vi "EnFlo_Tun_Heater_Control.vi"(1 "Heaters Enabled time (s)":dbl, 2 "Heaters Just Enabled":bool, 3 "Ch Names":string[](array[string]), 4 "Values":dbl[](array[numeric]) format="%.2f") -> (0 "Error String":string)   [LabVIEW 2021]
uses:
  ADAM Client/Sub VIs/ADAM Controls/Search_mode.ctl
  <vilib>/Analysis/baseanly.llb/Mean (DBL).vi
  ADAM_Global.vi
  Anemometry/Anemometry Sub Vis/Globals/EnFlo_Tunnel_Global.vi
  <vilib>/Analysis/NI_AALPro.lvlib
  <vilib>/Analysis/NI_AALBase.lvlib
panel:
  in  "Time (s) before killing heaters when exceeding max power":i32=350
  out "Heater State Happy":bool
  out "Error":dbl(graph)
  out "Derivative":dbl(graph)
  out "Integral":dbl(graph)
  out "Proportional":dbl(graph)
  out "Upper limit on Power":dbl
  in  "Proportional Error Deadband":dbl=0.03
  out "Read Values OK":bool
  out "History Out":dbl[](array[numeric])
  out "Current Temp":dbl
  out "Setpoint":dbl
  in  "Index To Display":i32
  out "Feedback Temperature":string
  in  "Minimum Power Change in %":dbl=0.05
  in  "Total History":i32=450
  out "Control Sum":dbl format="%#.1f"
  in  "Derivative History":i32=60
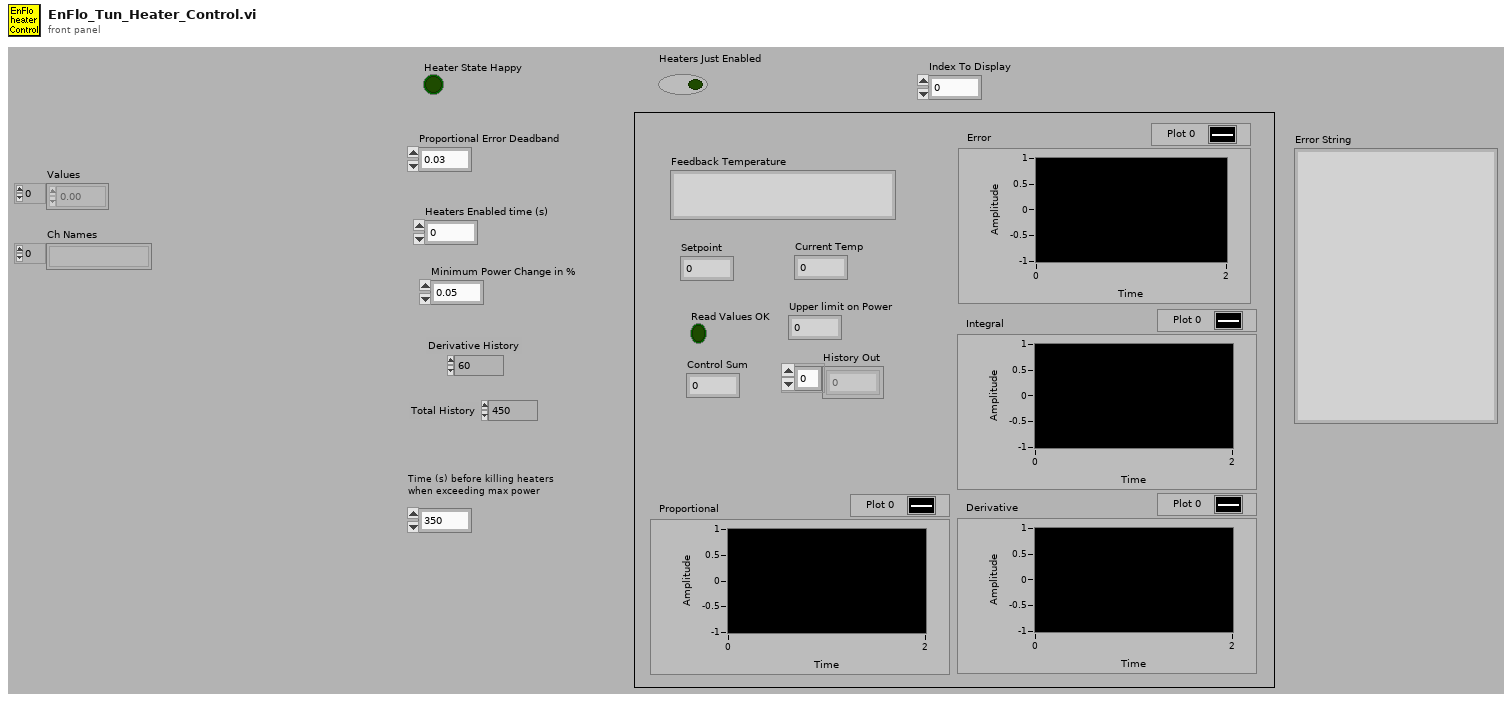
[diagram p1: front panel]
types:
  T1 = enum16{"On", "Off", "Always On", "Always Off", "Delete"}
  T2 = typedef "Search_mode.ctl" = enum16{"Between times", "All Times"}
  T3 = typedef "Ch_description_ADAM.ctl" = cluster{"Ch Name":string, "Type":T4, "Function":T5, "Ch State":T6, "Calibration type":T7, "A":dbl, "B":dbl, "C":dbl, "D":dbl, "Comments":string, "Address":T8, "String":string, "Duty":u16}
  T4 = typedef "Module_type_ADAM.ctl" = string
  T5 = typedef "Function_ADAM.ctl" = enum16{"Analogue Input", "Digital Input", "Event counter", "Event rate", "Analogue Output", "Digital Output", "Relay Output"}
  T6 = typedef "Channel_State.ctl" = enum16{"On", "Off", "Always On", "Always Off"}
  T7 = typedef "Calib_type_ADAM.ctl" = string
  T8 = typedef "Address.ctl" = cluster{"Main":i32, "Ch.":i32, "Sub":i32, "Port Name":string}
  T9 = cluster{"Bus Bar":string, "Connected Items":string[]}
  T10 = cluster{"Bus Bar":string, "Connected Items":string[]}[]
  T11 = cluster{"Centre Times":dbl[], "Output array":dbl[]}
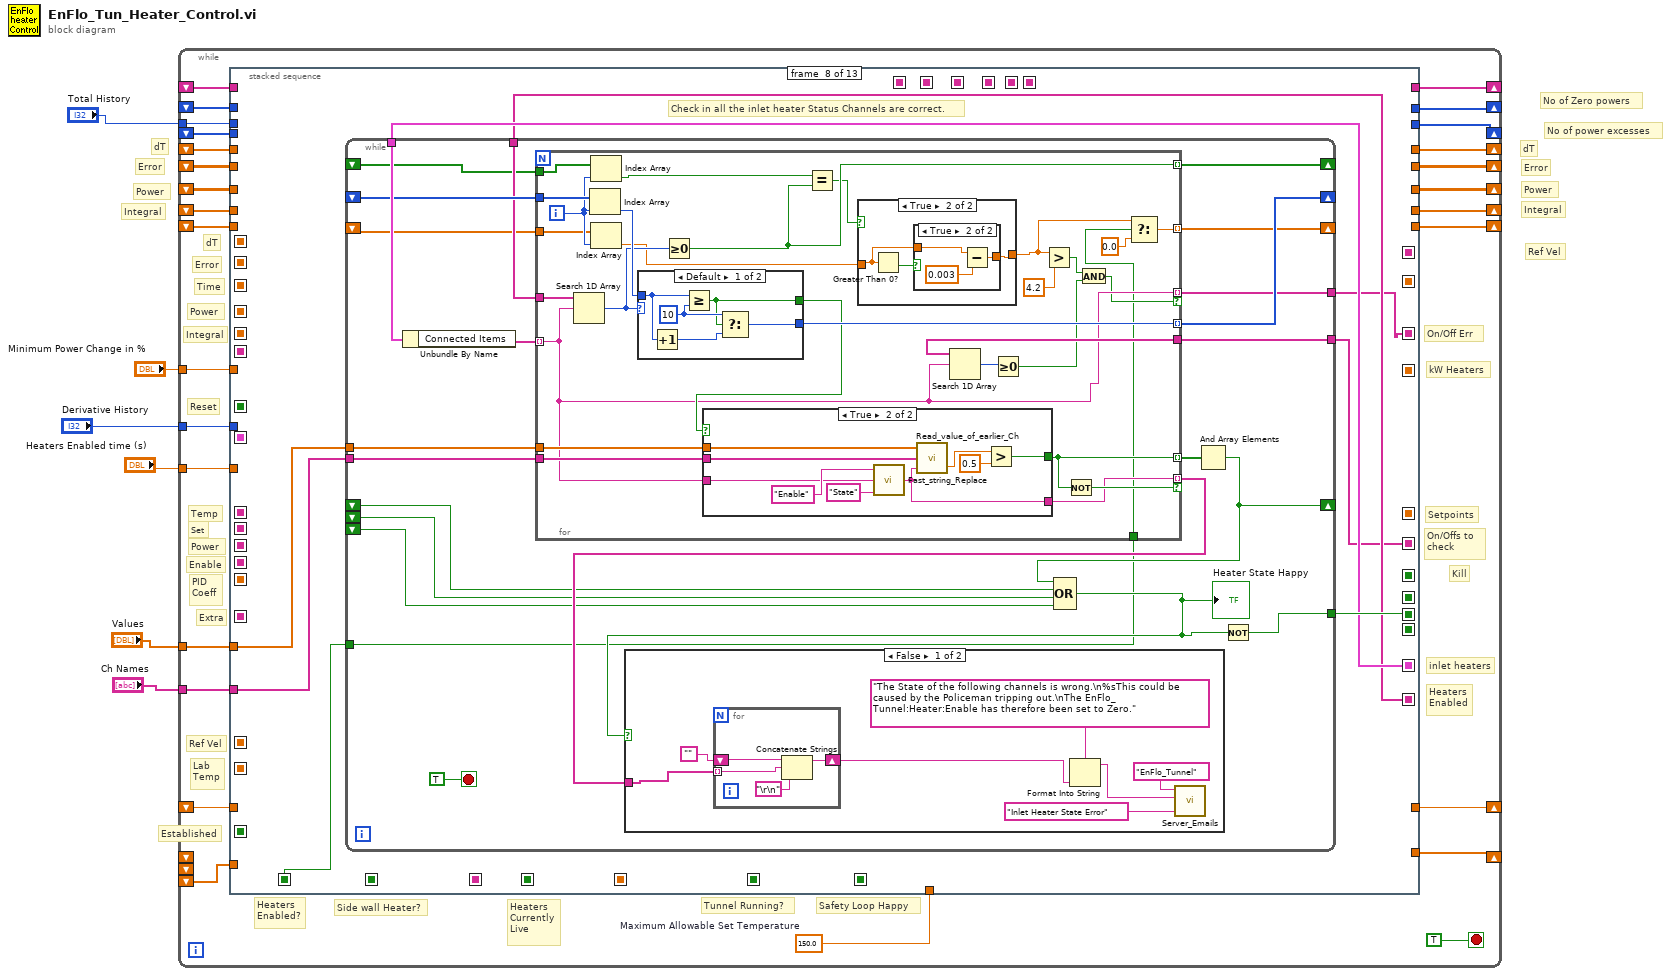
[diagram p0: block diagram]
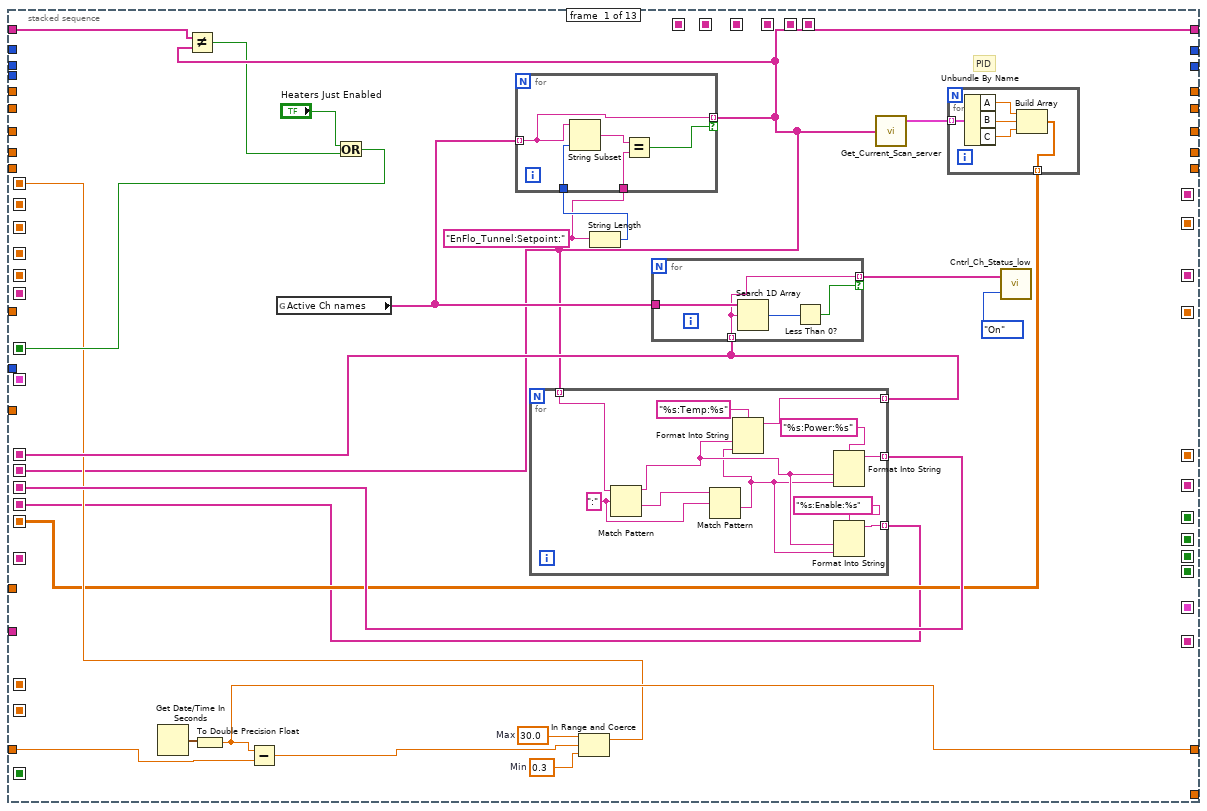
[diagram p2: hidden frame]
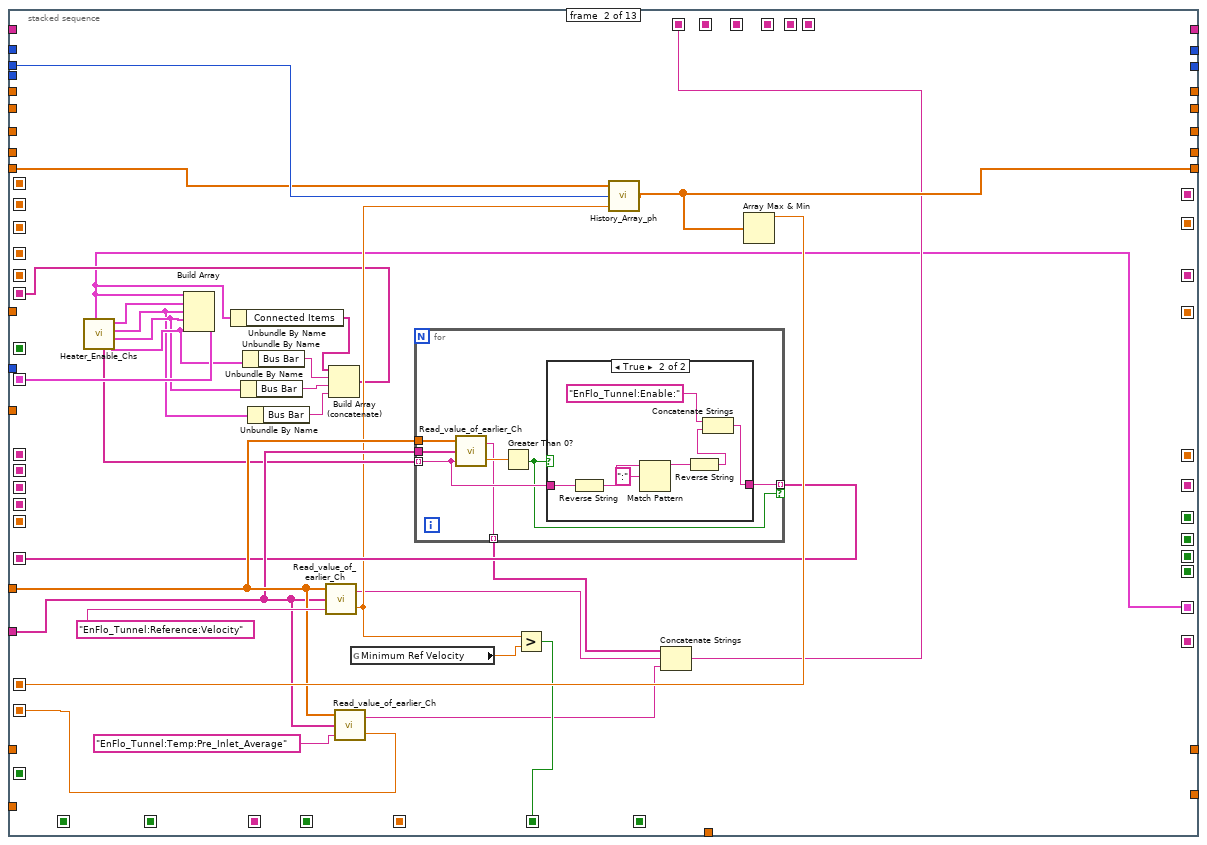
[diagram p3: hidden frame]
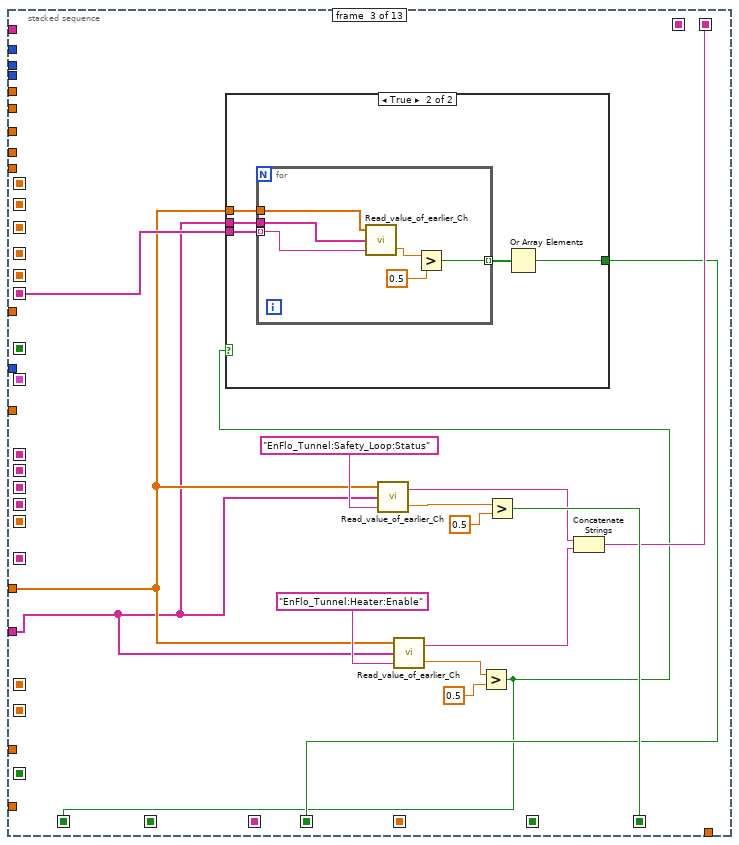
[diagram p5: hidden frame]
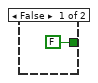
[diagram p6: hidden frame]
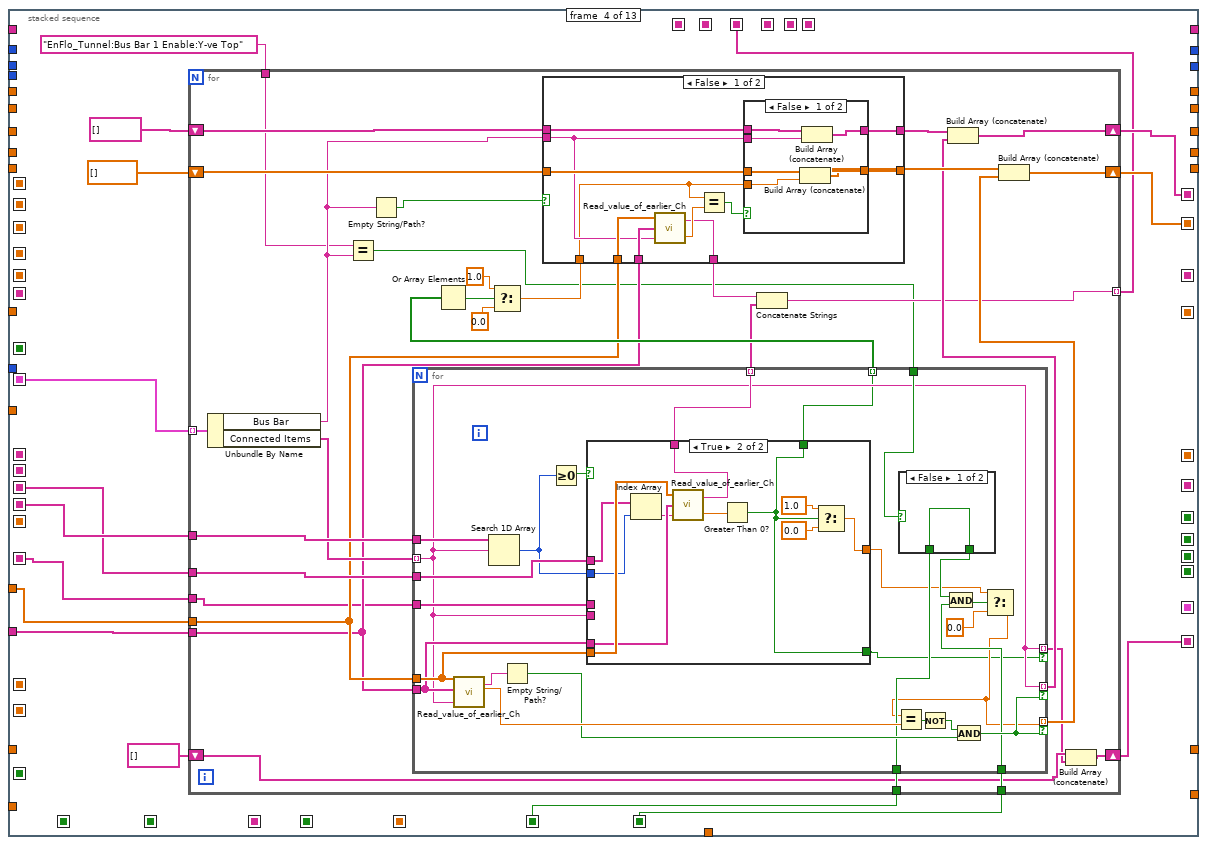
[diagram p7: hidden frame]
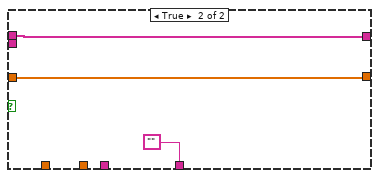
[diagram p9: hidden frame]
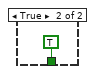
[diagram p10: hidden frame]
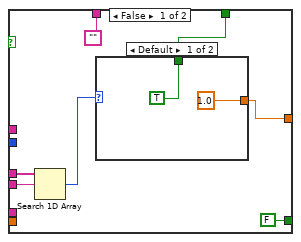
[diagram p11: hidden frame]
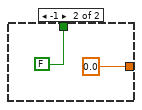
[diagram p12: hidden frame]
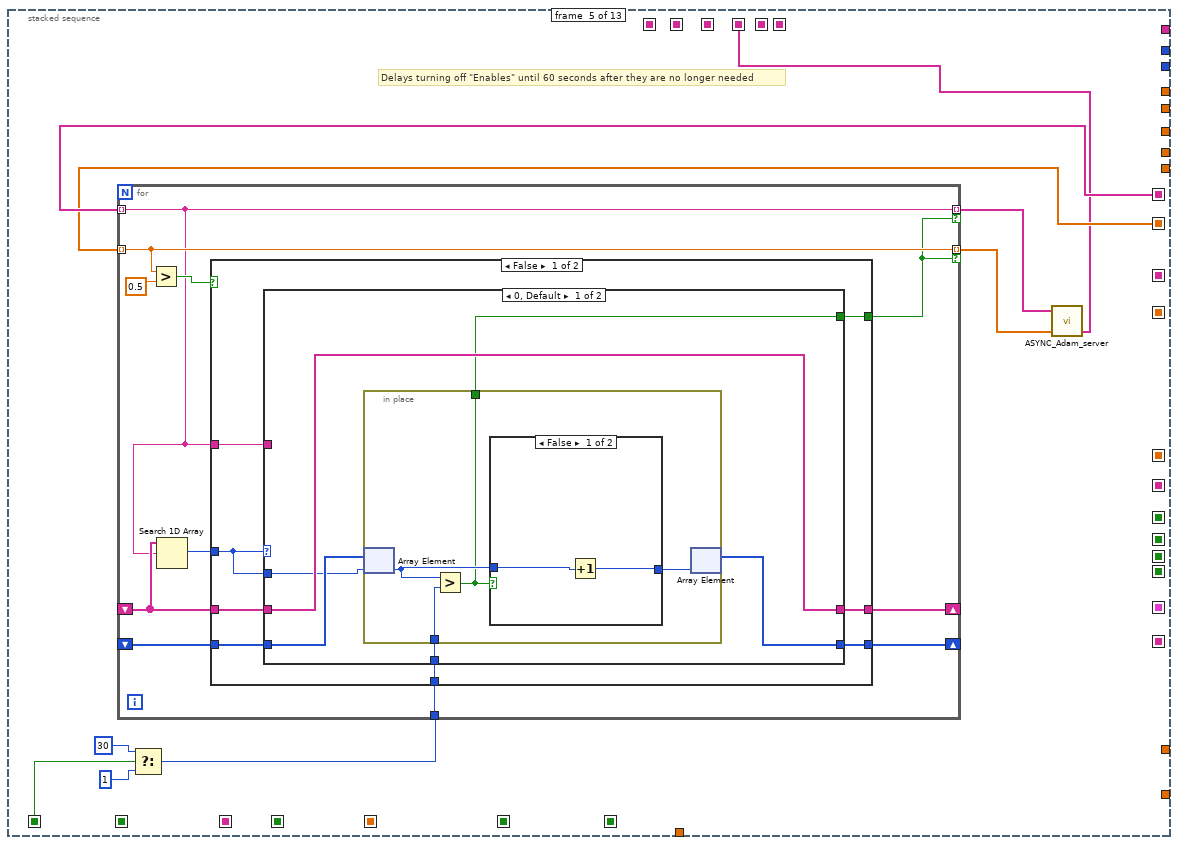
[diagram p13: hidden frame]
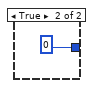
[diagram p14: hidden frame]
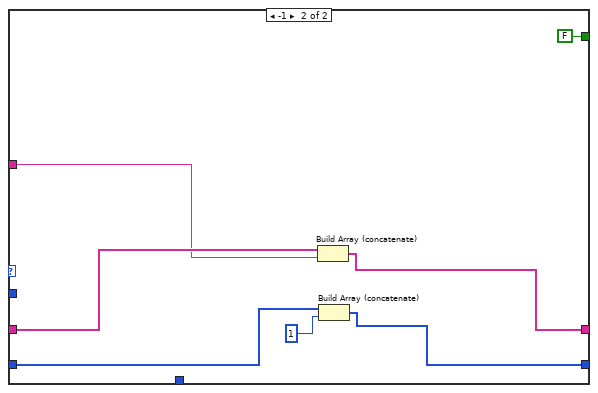
[diagram p15: hidden frame]
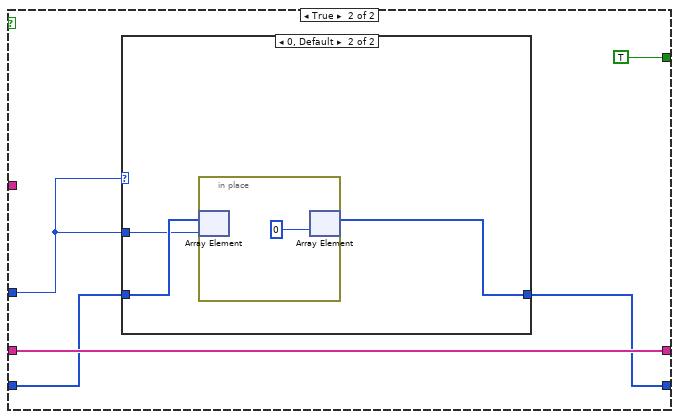
[diagram p16: hidden frame]
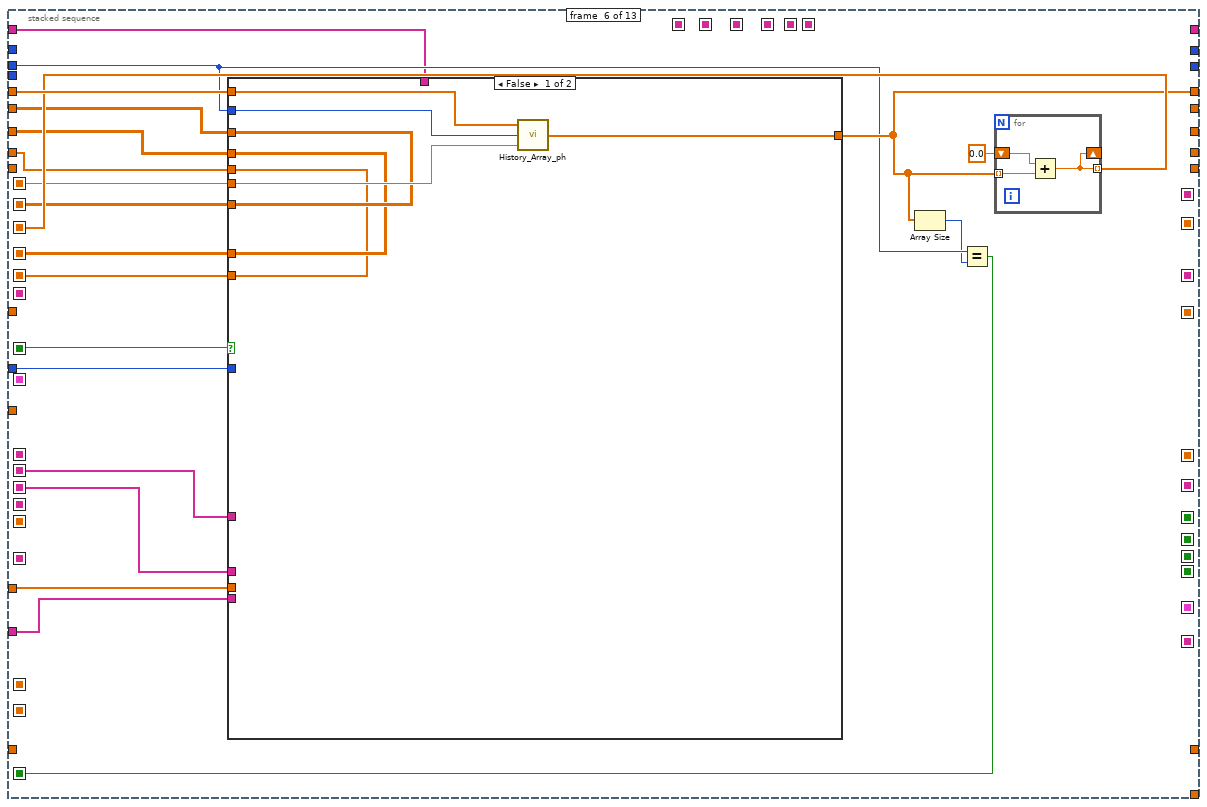
[diagram p18: hidden frame]
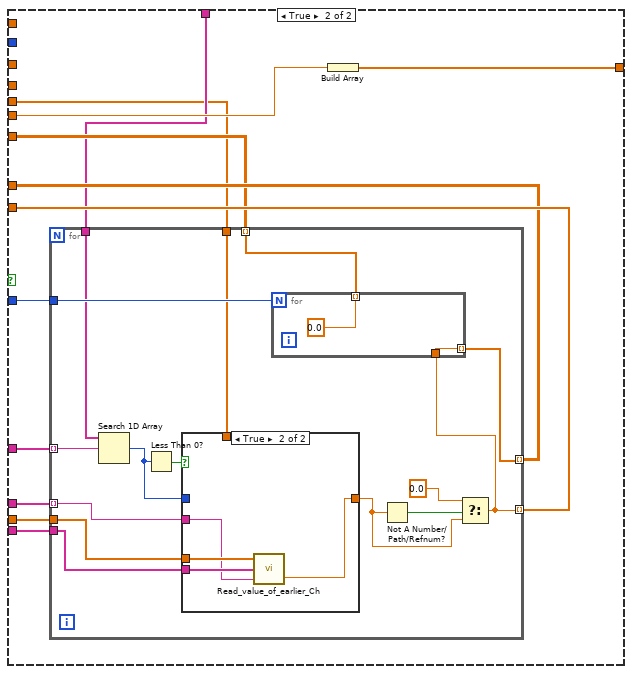
[diagram p19: hidden frame]
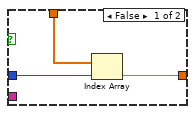
[diagram p20: hidden frame]
diagram:
  # "Established"
  # "No of Zero powers"
  # "No of power excesses"
  # "Ref Vel"
  # "Integral"
  # "Power"
  # "Error"
  # "dT"
  # "Power"
  # "Integral"
  # "Error"
  # "dT"
  n1 = while {
    shift-right: [w32] -> _
    shift-left: _ -> [w33]
    shift-right: [w28] -> _
    shift-left: _ -> [w31]
    shift-right: [w30] -> _
    shift-left: _ -> [w29]
    shift-right: [w26] -> _
    shift-left: _ -> [w27]
    shift-right: [w24] -> _
    shift-left: _ -> [w25]
    tunnel: "Total History" -> [w23]
    tunnel: "Ch Names" -> [w21]
    tunnel: "Values" -> [w20]
    tunnel: "Minimum Power Change in %" -> [w19]
    shift-right: [w18] -> _
    shift-left: _ -> [_]
    shift-left: _ -> [_]
    tunnel: "Heaters Enabled time (s)" -> [w17]
    shift-right: [w15] -> _
    shift-left: _ -> [w16]
    shift-right: [w14] -> _
    shift-left: _ -> [w13]
    shift-right: [w11] -> _
    shift-left: _ -> [w12]
    shift-right: [w10] -> _
    shift-left: _ -> [w9]
    shift-left: _ -> [w8]
    tunnel: "Derivative History" -> [w7]
    stop <- TRUE stop-if-true
    w22 = 150.0  # Maximum Allowable Set Temperature
    # "On/Offs to\ncheck"
    # "On/Off Err"
    # "kW Heaters"
    # "inlet heaters"
    # "Heaters\nEnabled"
    # "Heaters\nCurrently\nLive"
    # "Heaters\nEnabled?"
    # "Safety Loop Happy"
    # "Tunnel Running?"
    # "Setpoints"
    # "Extra"
    # "Enable"
    # "Side wall Heater?"
    # "Lab\nTemp"
    # "Ref Vel"
    # "PID\nCoeff"
    # "dT"
    # "Integral"
    # "Power"
    # "Error"
    # "Reset"
    # "Kill"
    # "Power"
    # "Set"
    # "Temp"
    # "Time"
    n2 = stacked-sequence {
      seq-local: [_ _ _ _ _ w347 _ _ _ _ _ _ _] -> [_ _ _ _ _ _ w433 _ w812 _ _ _ _]
      seq-local: [w47 _ _ _ _ _ _ _ _ _ _ _ _] -> [_ _ _ _ _ _ w430 _ _ _ _ w1028 _]
      seq-local: [w37 _ _ _ _ _ _ _ _ _ _ _ _] -> [_ _ _ _ _ w330 w429 _ _ _ _ w1027 _]
      seq-local: [w54 _ _ _ _ _ _ _ _ _ _ _ _] -> [_ _ _ w165 _ w333 w428 _ _ _ _ w1030 _]
      seq-local: [_ _ _ _ _ _ w413 _ _ _ _ _ _] -> [_ _ _ _ _ _ _ _ w815 _ _ _ _]
      seq-local: [_ _ _ _ _ _ _ _ w814 _ _ _ _] -> [_ _ _ _ _ _ _ _ _ _ _ _ w1110]
      seq-local: [_ _ _ _ _ _ _ _ _ _ w954 _ _] -> [_ _ _ _ _ _ _ _ _ _ _ _ w1111]
      seq-local: [w42 _ _ _ _ _ _ _ _ _ _ _ _] -> [_ _ _ _ _ w346 w424 _ _ _ _ _ _]
      seq-local: [w43 _ _ _ _ _ _ _ _ _ _ _ _] -> [_ _ _ _ _ w349 _ _ _ _ _ w1013 _]
      seq-local: [_ _ _ _ _ w345 _ _ _ _ _ _ _] -> [_ _ _ _ _ _ w421 _ _ _ _ _ _]
      seq-local: [_ _ _ _ _ w343 _ _ _ _ _ _ _] -> [_ _ _ _ _ _ w422 _ _ _ _ _ _]
      seq-local: [_ _ _ _ _ w341 _ _ _ _ _ _ _] -> [_ _ _ _ _ _ w423 _ _ _ _ _ _]
      seq-local: [w40 _ _ _ _ _ _ _ _ _ _ _ _] -> [_ _ _ _ _ _ w419 _ _ _ _ _ _]
      seq-local: [_ _ _ _ _ w337 _ _ _ _ _ _ _] -> [_ _ _ _ _ _ _ _ _ _ _ w1007 _]
      seq-local: [_ w104 _ _ _ _ _ _ _ _ _ _ _] -> [_ _ _ _ _ _ w415 _ _ _ _ w1010 _]
      seq-local: [_ w108 _ _ _ _ _ _ _ _ _ _ _] -> [_ _ _ _ _ _ w414 _ _ _ _ _ _]
      seq-local: [_ _ _ _ _ _ w412 _ _ _ _ _ _] -> [_ _ _ _ _ _ _ _ w813 _ _ _ _]
      seq-local: [_ _ _ _ _ _ w411 _ _ _ _ _ _] -> [_ _ _ _ _ _ _ _ _ _ _ w1014 _]
      seq-local: [w38 _ _ _ _ _ _ _ _ _ _ _ _] -> [_ _ _ w166 _ _ w402 _ _ _ _ _ _]
      seq-local: [_ w103 _ _ _ _ _ _ _ _ _ _ _] -> [_ _ _ w162 _ _ _ _ _ _ _ _ _]
      seq-local: [_ w99 _ _ _ _ _ _ _ _ _ _ _] -> [_ _ _ w161 _ _ _ _ _ _ _ _ _]
      seq-local: [_ _ _ w160 _ _ _ _ _ _ _ _ _] -> [_ _ _ _ w280 _ _ _ _ _ _ _ _]
      seq-local: [_ _ _ w159 _ _ _ _ _ _ _ _ _] -> [_ _ _ _ w277 _ _ _ _ _ _ _ _]
      seq-local: [_ _ _ _ _ _ w408 _ _ _ _ _ _] -> [_ _ _ _ _ _ _ _ _ _ w951 _ _]
      seq-local: [_ w96 _ _ _ _ _ _ _ _ _ _ _] -> [_ _ _ w157 _ _ _ _ _ _ _ _ _]
      seq-local: [_ _ w137 _ _ _ _ _ _ _ _ _ _] -> [_ _ _ w156 _ _ _ _ _ _ _ _ _]
      seq-local: [_ w92 _ _ _ _ _ _ _ _ _ _ _] -> [_ _ _ _ _ _ _ _ _ _ _ _ w1115]
      seq-local: [_ _ w131 _ _ _ _ _ _ _ _ _ _] -> [_ _ _ _ _ _ _ _ _ _ _ _ w1116]
      seq-local: [_ _ _ w158 _ _ _ _ _ _ _ _ _] -> [_ _ _ _ _ _ _ _ _ _ _ _ w1117]
      seq-local: [_ _ _ _ w276 _ _ _ _ _ _ _ _] -> [_ _ _ _ _ _ _ _ _ _ _ _ w1118]
      seq-local: [_ _ _ _ _ _ w407 _ _ _ _ _ _] -> [_ _ _ _ _ _ _ _ _ _ _ _ w1119]
      seq-local: [_ _ _ _ _ _ _ _ _ _ _ w1005 _] -> [_ _ _ _ _ _ _ _ _ _ _ _ w1120]
      seq-local: [_ _ w126 _ _ _ _ _ _ _ _ _ _] -> [_ _ _ _ w275 _ w406 w711 w810 _ _ w1004 _]
      seq-local: [_ w84 _ _ _ _ _ _ _ _ _ _ _] -> [_ _ w130 _ _ _ _ _ _ _ _ _ _]
      seq-local: [_ _ w127 _ _ _ _ _ _ _ _ _ _] -> [_ _ _ _ _ _ _ _ _ w934 w949 _ _]
      seq-local: [_ _ _ w153 _ _ _ _ _ _ _ _ _] -> [_ _ _ _ _ _ _ w714 _ _ _ _ _]
      seq-local: [_ _ _ _ _ _ _ w716 _ _ _ _ _] -> [_ _ _ _ _ _ _ _ _ _ _ _ w1112]
      seq-local: [_ w82 _ _ _ _ _ _ _ _ _ _ _] -> [_ _ _ _ _ _ _ w715 _ _ _ _ _]
      seq-local: [_ _ _ _ _ _ _ w713 _ _ _ _ _] -> [_ _ _ _ _ _ _ _ _ w937 _ _ _]
      seq-local: [_ _ _ _ _ _ _ _ _ w933 _ _ _] -> [_ _ _ _ _ _ _ _ _ _ _ _ w1108]
      seq-local: [_ _ _ _ _ _ w404 _ _ _ _ _ _] -> [_ _ _ _ _ _ _ _ _ _ _ _ w1106]
      seq-local: [_ _ _ _ _ _ w403 _ _ _ _ _ _] -> [_ _ _ _ _ _ _ w712 _ _ _ _ _]
      tunnel: w33 -> [_ _ _ _ _ w350 w401 _ _ _ _ _ _]
      tunnel: [_ _ _ _ _ w339 _ _ _ _ _ _ _] -> w32
      tunnel: w31 -> [_ _ _ _ _ w344 _ _ _ _ _ _ _]
      tunnel: [w48 _ _ _ _ _ _ _ _ _ _ _ _] -> w30
      tunnel: w29 -> [w50 _ _ _ _ _ _ _ _ _ _ _ _]
      tunnel: [_ _ _ _ _ _ w434 _ _ _ _ _ _] -> w28
      tunnel: w27 -> [_ _ _ _ _ w342 _ _ _ _ _ w1029 _]
      tunnel: [_ _ _ _ _ _ w432 _ _ _ _ _ _] -> w26
      tunnel: w25 -> [_ _ _ _ _ w340 _ _ _ _ _ _ _]
      tunnel: [_ _ _ _ _ _ w431 _ _ _ _ _ _] -> w24
      tunnel: w23 -> [_ w107 _ _ _ w338 w425 _ w816 _ w955 _ _]
      tunnel: w22 -> [_ _ _ _ _ _ _ _ _ _ w950 _ _]
      tunnel: w21 -> [_ w101 w128 w167 _ w334 w427 w717 _ _ w953 w1025 w1121]
      tunnel: w20 -> [_ w102 w129 w168 _ w335 w426 w718 _ _ w952 w1026 _]
      tunnel: w19 -> [_ _ _ _ _ _ w420 _ _ _ _ w1022 _]
      tunnel: [_ _ _ _ _ _ _ _ _ _ _ w1016 _] -> w18
      tunnel: w8 -> [_ _ _ _ _ _ _ _ _ _ _ w1015 _]
      tunnel: w17 -> [_ _ _ _ _ _ w418 _ _ _ _ _ _]
      tunnel: w16 -> [_ w106 _ _ _ _ _ _ _ _ _ _ _]
      tunnel: [_ w105 _ _ _ _ _ _ _ _ _ _ _] -> w15
      tunnel: [_ _ _ _ _ _ w410 _ _ _ _ _ _] -> w14
      tunnel: w13 -> [_ _ _ _ _ _ w409 _ _ _ _ _ _]
      tunnel: w12 -> [_ _ _ _ _ _ _ _ _ _ _ w1012 _]
      tunnel: [_ _ _ _ _ _ _ _ _ _ _ w1011 _] -> w11
      tunnel: [w37 _ _ _ _ _ _ _ _ _ _ _ _] -> w10
      tunnel: w9 -> [w35 _ _ _ _ w331 _ _ _ _ _ _ _]
      tunnel: w7 -> [_ _ _ _ _ w332 w405 _ _ _ _ _ _]
      frame #0 {
        w52 = 0.3  # Min
        w51 = 30.0  # Max
        w55 = "EnFlo_Tunnel:Setpoint:"
        # "PID"
        n3 = Get Date/Time In Seconds() -> (seconds since 1Jan1904=w53:timestamp)
        n4 = To Double Precision Float(number=w53) -> (double precision float=w48:dbl)
        n5 = Subtract(x=w48, y=w50) -> (x-y=w49:dbl)
        n6 = global read "ADAM_Global.vi" "Active Ch names"() -> (w45:string[])
        n7 = In Range and Coerce(upper limit=w51, x=w49, lower limit=w52) -> (coerced(x)=w42:dbl)  [unwired: 1 out]
        n8 = String Length(string=w55) -> (length=w56:i32)
        n9 = for {
          tunnel: w45 -> [w67] mode=indexing
          tunnel: w56 -> [w70]
          tunnel: w55 -> [w69]
          tunnel: [w67] -> w37 mode=indexing if=w66
          n10 = String Subset(string=w67, length (rest)=w70) -> (substring=w68:string)  [unwired: 1 out]
          n11 = Equal?(x=w68, y=w69) -> (x = y?=w66:bool)
        }
        n12 = Not Equal?(x=w35, y=w37) -> (x != y?=w36:bool)
        n13 = Or(x="Heaters Just Enabled", y=w36) -> (x .or. y?=w43:bool)
        n14 = for {
          tunnel: w37 -> [w75] mode=indexing
          tunnel: [w76] -> w54 mode=indexing
          tunnel: [w77] -> w47 mode=indexing
          tunnel: [w71] -> w38 mode=indexing
          w80 = ":" ("regular expression")
          n15 = Match Pattern(string=w75, regular expression=w80) -> (before substring=w73:string, after substring=w81:string)  [unwired: 3 out]
          n16 = Match Pattern(string=w81, regular expression=w80) -> (after substring=w72:string)  [unwired: 4 out]
          n17 = Format Into String(format string="%s:Temp:%s", w73, w72) -> (resulting string=w77:string)  [unwired: 2 in, 1 out]
          n18 = Format Into String(format string="%s:Power:%s", w73, w72) -> (resulting string=w76:string)  [unwired: 2 in, 1 out]
          n19 = Format Into String(format string="%s:Enable:%s", w73, w72) -> (resulting string=w71:string)  [unwired: 2 in, 1 out]
        }
        n20 = for {
          tunnel: w47 -> [w64] mode=indexing
          tunnel: w45 -> [w65]
          tunnel: [w64] -> w39 mode=indexing if=w62
          n21 = Search 1D Array(1D array=w65, element=w64) -> (index of element=w63:i32)  [unwired: 1 in]
          n22 = Less Than 0?(x=w63) -> (x < 0?=w62:bool)
        }
        n23 = call "Get_Current_Scan_server.vi"("Desired Channels"=w37) -> ("Ch Description Array"=w41:T3[])  [unwired: 2 out]
        n24 = for {
          tunnel: w41 -> [w61] mode=indexing
          tunnel: [w57] -> w40 mode=indexing
          n25 = Unbundle By Name(w61) -> ("A"=w60:dbl, "B"=w59:dbl, "C"=w58:dbl)
          n26 = Build Array(w60, w59, w58) -> (w57:dbl[])
        }
        n27 = call "Cntrl_Ch_Status_low.vi"("Mode"=T1."On", "Channel names"=w39) -> ()  [unwired: 1 out]
      }
      frame #1 {
        n28 = call "Heater_Enable_Chs.vi"() -> ("Bus Bar 4"=w90:T9, "Bus Bar 3"=w89:T9, "Bus Bar 2"=w88:T9, "Bus Bar 1"=w91:T9, "Wanted if these channels are great than zero"=w100:string[], "Inlet Heaters"=w82:T9)  [unwired: 4 in]
        n29 = Build Array(w82, w91, w88, w89, w90) -> (w103:T10)
        n30 = Unbundle By Name(w82) -> ("Connected Items"=w83:string[])
        n31 = Unbundle By Name(w89) -> ("Bus Bar"=w86:string)
        n32 = Unbundle By Name(w90) -> ("Bus Bar"=w87:string)
        n33 = Unbundle By Name(w88) -> ("Bus Bar"=w85:string)
        n34 = call "Read_value_of_earlier_Ch.vi"("Desired Ch to Read"="EnFlo_Tunnel:Reference:Velocity", "Ch names"=w101, "Present scan array"=w102) -> ("Value"=w97:dbl, "Scan comment"=w94:string)  [unwired: 1 in]
        n35 = Build Array (concatenate)(w83, w87, w86, w85) -> (w84:string[])
        n36 = call "Read_value_of_earlier_Ch.vi"("Desired Ch to Read"="EnFlo_Tunnel:Temp:Pre_Inlet_Average", "Ch names"=w101, "Present scan array"=w102) -> ("Value"=w108:dbl, "Scan comment"=w93:string)  [unwired: 1 in]
        n37 = global read "EnFlo_Tunnel_Global.vi" "Minimum Ref Velocity"() -> (w98:dbl)
        n38 = for {
          tunnel: w102 -> [w117]
          tunnel: w101 -> [w116]
          tunnel: w100 -> [w114] mode=indexing
          tunnel: [w113] -> w99 mode=indexing if=w112
          tunnel: [w111] -> w95 mode=indexing
          n39 = call "Read_value_of_earlier_Ch.vi"("Desired Ch to Read"=w114, "Ch names"=w116, "Present scan array"=w117) -> ("Value"=w115:dbl, "Scan comment"=w111:string)  [unwired: 1 in]
          n40 = Greater Than 0?(x=w115) -> (x > 0?=w112:bool)
          n41 = case shown="True" w112 {
            tunnel: w114 -> [w118 w125]
            tunnel: [w118 w119] -> w113
            frame False {
            }
            frame True {
              n42 = Reverse String(1:w125) -> (0:w124:string)
              n43 = Match Pattern(string=w124, regular expression=":") -> (before substring=w122:string)  [unwired: 1 in, 3 out]
              n44 = Reverse String(1:w122) -> (0:w120:string)
              n45 = Concatenate Strings("EnFlo_Tunnel:Enable:", w120) -> (w119:string)
            }
          }
        }
        n46 = Greater?(x=w97, y=w98) -> (0:w96:bool)
        n47 = call "History_Array_ph.vi"("Current Value"=w97, "Desired Length"=w107, "History In"=w106) -> ("History Out"=w105:dbl[])
        n48 = Concatenate Strings(w95, w94, w93) -> (w92:string)
        n49 = Array Max & Min(array=w105) -> (max value=w104:dbl)  [unwired: 3 out]
      }
      frame #2 {
        n50 = call "Read_value_of_earlier_Ch.vi"("Desired Ch to Read"="EnFlo_Tunnel:Safety_Loop:Status", "Ch names"=w128, "Present scan array"=w129) -> ("Value"=w140:dbl, "Scan comment"=w133:string)  [unwired: 1 in]
        n51 = call "Read_value_of_earlier_Ch.vi"("Desired Ch to Read"="EnFlo_Tunnel:Heater:Enable", "Ch names"=w128, "Present scan array"=w129) -> ("Value"=w134:dbl, "Scan comment"=w132:string)  [unwired: 1 in]
        n52 = Greater?(x=w134, y=0.5) -> (0:w126:bool)
        n53 = case shown="True" w126 {
          tunnel: w130 -> [_ w146]
          tunnel: w129 -> [_ w145]
          tunnel: w128 -> [_ w144]
          tunnel: [FALSE w142] -> w127
          frame False {
          }
          frame True {
            n54 = for {
              tunnel: w146 -> [w152] mode=indexing
              tunnel: w145 -> [w151]
              tunnel: w144 -> [w150]
              tunnel: [w147] -> w143 mode=indexing
              n55 = call "Read_value_of_earlier_Ch.vi"("Desired Ch to Read"=w152, "Ch names"=w150, "Present scan array"=w151) -> ("Value"=w149:dbl)  [unwired: 1 in, 1 out]
              n56 = Greater?(x=w149, y=0.5) -> (0:w147:bool)
            }
            n57 = Or Array Elements(Boolean array=w143) -> (logical OR=w142:bool)
          }
        }
        n58 = Greater?(x=w140, y=0.5) -> (0:w137:bool)
        n59 = Concatenate Strings(w133, w132) -> (w131:string)
      }
      frame #3 {
        n60 = for {
          tunnel: w168 -> [w183]
          tunnel: w167 -> [w182]
          tunnel: w166 -> [w200]
          tunnel: w165 -> [w199]
          tunnel: w162 -> [w197] mode=indexing
          shift-right: [w194] -> w160
          shift-left: string[] [] -> [w196]
          shift-right: [w193] -> w159
          shift-left: dbl[] [] -> [w191]
          tunnel: w161 -> [w181]
          tunnel: [w178] -> w158 mode=indexing
          tunnel: w157 -> [w177]
          tunnel: w156 -> [w176]
          tunnel: "EnFlo_Tunnel:Bus Bar 1 Enable:Y-ve Top" -> [w174]
          shift-right: [w169] -> w153
          shift-left: string[] [] -> [w171]
          n61 = Unbundle By Name(w197) -> ("Bus Bar"=w175:string, "Connected Items"=w198:string[])
          n62 = Equal?(x=w174, y=w175) -> (x = y?=w172:bool)
          n63 = Empty String/Path?(string/path=w175) -> (empty?=w173:bool)
          n64 = for {
            tunnel: w183 -> [w244]
            tunnel: w182 -> [w243]
            tunnel: w198 -> [w225] mode=indexing
            tunnel: w200 -> [w247]
            tunnel: [w227] -> w190 mode=indexing if=w236
            tunnel: [w225] -> w186 mode=indexing if=w236
            tunnel: w199 -> [w242]
            tunnel: [w224] -> w185 mode=indexing
            tunnel: w181 -> [w235]
            tunnel: [w234] -> w179 mode=indexing
            tunnel: w177 -> [w233]
            tunnel: w176 -> [w231]
            tunnel: w172 -> [w226]
            tunnel: [w225] -> w170 mode=indexing if=w223
            n65 = call "Read_value_of_earlier_Ch.vi"("Desired Ch to Read"=w225, "Ch names"=w243, "Present scan array"=w244) -> ("Value"=w246:dbl, "Scan comment"=w240:string)  [unwired: 1 in]
            n66 = Search 1D Array(1D array=w247, element=w225) -> (index of element=w241:i32)  [unwired: 1 in]
            n67 = Empty String/Path?(string/path=w240) -> (empty?=w238:bool)
            n68 = Greater Or Equal To 0?(x=w241) -> (x >= 0?=w237:bool)
            n69 = case shown="True" w237 {
              tunnel: [w256 w264] -> w228
              tunnel: w244 -> [_ w271]
              tunnel: w243 -> [_ w270]
              tunnel: w242 -> [_ w269]
              tunnel: w241 -> [_ w268]
              tunnel: [w255 w261] -> w224
              tunnel: w235 -> [w254 _]
              tunnel: w225 -> [w253 _]
              tunnel: ["" w263] -> w234
              tunnel: [FALSE w261] -> w223
              frame False {
                n70 = Search 1D Array(1D array=w254, element=w253) -> (index of element=w252:i32)  [unwired: 1 in]
                n71 = case shown="Default" w252 {
                  tunnel: [1.0 0.0] -> w256
                  tunnel: [TRUE FALSE] -> w255
                  frame Default {
                  }
                  frame -1 {
                  }
                }
              }
              frame True {
                n72 = Index Array(array=w269, index=w268) -> (element=w267:string)
                n73 = call "Read_value_of_earlier_Ch.vi"("Desired Ch to Read"=w267, "Ch names"=w270, "Present scan array"=w271) -> ("Value"=w262:dbl, "Scan comment"=w263:string)  [unwired: 1 in]
                n74 = Greater Than 0?(x=w262) -> (x > 0?=w261:bool)
                n75 = Select(t=1.0, s=w261, f=0.0) -> (s? t:f=w264:dbl)
              }
            }
            n76 = case shown="False" w226 {
              tunnel: [w248 TRUE] -> w232
              tunnel: w233 -> [w248 _]
              frame False {
              }
              frame True {
              }
            }
            n77 = And(x=w232, y=w231) -> (x .and. y?=w229:bool)
            n78 = Select(t=w228, s=w229, f=0.0) -> (s? t:f=w227:dbl)
            n79 = Equal?(x=w227, y=w246) -> (x = y?=w245:bool)
            n80 = Not(x=w245) -> (.not. x?=w239:bool)
            n81 = And(x=w239, y=w238) -> (x .and. y?=w236:bool)
          }
          n82 = Or Array Elements(Boolean array=w185) -> (logical OR=w184:bool)
          n83 = Select(t=1.0, s=w184, f=0.0) -> (s? t:f=w187:dbl)
          n84 = case shown="False" w173 {
            tunnel: w196 -> [w211 w222]
            tunnel: w175 -> [w205 _]
            tunnel: [w210 w222] -> w195
            tunnel: [w209 w221] -> w192
            tunnel: w191 -> [w208 w221]
            tunnel: w187 -> [w203 _]
            tunnel: w183 -> [w207 _]
            tunnel: w182 -> [w206 _]
            tunnel: [w201 ""] -> w180
            frame False {
              n85 = call "Read_value_of_earlier_Ch.vi"("Desired Ch to Read"=w205, "Ch names"=w206, "Present scan array"=w207) -> ("Value"=w202:dbl, "Scan comment"=w201:string)  [unwired: 1 in]
              n86 = Equal?(x=w203, y=w202) -> (x = y?=w204:bool)
              n87 = case shown="False" w204 {
                tunnel: w211 -> [w217 w219]
                tunnel: [w216 w219] -> w210
                tunnel: [w215 w218] -> w209
                tunnel: w208 -> [w214 w218]
                tunnel: w203 -> [w213 _]
                tunnel: w205 -> [w212 _]
                frame False {
                  n88 = Build Array (concatenate)(w214, w213) -> (w215:dbl[])
                  n89 = Build Array (concatenate)(w217, w212) -> (w216:string[])
                }
                frame True {
                }
              }
            }
            frame True {
            }
          }
          n90 = Concatenate Strings(w180, w179) -> (w178:string)
          n91 = Build Array (concatenate)(w195, w186) -> (w194:string[])
          n92 = Build Array (concatenate)(w192, w190) -> (w193:dbl[])
          n93 = Build Array (concatenate)(w171, w170) -> (w169:string[])
        }
      }
      frame #4 {
        # "Delays turning off \"Enables\" until 60 seconds after they are no longer needed"
        n94 = Select(t=30 ("y"), s=w275, f=1 ("y")) -> (s? t:f=w272:i32)
        n95 = for {
          tunnel: [w283] -> w279 mode=indexing if=w282
          tunnel: w280 -> [w283] mode=indexing
          tunnel: [w291] -> w278 mode=indexing if=w282
          tunnel: w277 -> [w291] mode=indexing
          shift-right: [w285] -> _
          shift-left: _ -> [w286]
          shift-right: [w284] -> _
          shift-left: _ -> [w287]
          tunnel: w272 -> [w281]
          n96 = Greater?(x=w291, y=0.5) -> (0:w289:bool)
          n97 = Search 1D Array(1D array=w287, element=w283) -> (index of element=w288:i32)  [unwired: 1 in]
          n98 = case shown="False" w289 {
            tunnel: w288 -> [w294 w321]
            tunnel: w287 -> [w299 w324]
            tunnel: w286 -> [w298 w322]
            tunnel: [w297 w323] -> w285
            tunnel: [w296 w324] -> w284
            tunnel: w283 -> [w295 _]
            tunnel: [w293 TRUE] -> w282
            tunnel: w281 -> [w292 _]
            frame False {
              n99 = case shown="0, Default" w294 {
                tunnel: w299 -> [w303 w319]
                tunnel: w298 -> [w305 w318]
                tunnel: [w304 w317] -> w297
                tunnel: [w303 w316] -> w296
                tunnel: w295 -> [_ w315]
                tunnel: w294 -> [w301 _]
                tunnel: [w302 FALSE] -> w293
                tunnel: w292 -> [w300 _]
                frame 0, Default {
                  n100 = in-place {
                    in-place-border: [w307] -> w302
                    in-place-border: w300 -> [w306]
                    n101 = in-place-array #1(w305, w301) -> (w308:i32)
                    n102 = Greater?(x=w308, y=w306) -> (0:w307:bool)
                    n103 = case shown="False" w307 {
                      tunnel: [w310 0] -> w309
                      tunnel: w308 -> [w311 _]
                      frame False {
                        n104 = Increment(x=w311) -> (x+1=w310:i32)
                      }
                      frame True {
                      }
                    }
                    n105 = in-place-array #1(w309) -> (w304:i32[])  [unwired: 1 out]
                  }
                }
                frame -1 {
                  n106 = Build Array (concatenate)(w319, w315) -> (w316:string[])
                  n107 = Build Array (concatenate)(w318, 1) -> (w317:i32[])
                }
              }
            }
            frame True {
              n108 = case shown="0, Default" w321 {
                tunnel: [w325 w326] -> w323
                tunnel: w322 -> [w325 w328]
                tunnel: w321 -> [_ w327]
                frame -1 {
                }
                frame 0, Default {
                  n109 = in-place {
                    n110 = in-place-array #2(w328, w327) -> ()  [unwired: 1 out]
                    n111 = in-place-array #2(0) -> (w326:i32[])  [unwired: 1 out]
                  }
                }
              }
            }
          }
        }
        n112 = call "ASYNC_Adam_server.vi"("Values"=w278, "Channel Names"=w279) -> ("Scan Comments"=w276:string[])  [unwired: 1 in, 2 out]
      }
      frame #5 {
        n113 = case shown="False" w349 {
          tunnel: [w360 w372] -> w339
          tunnel: w350 -> [w359 _]
          tunnel: w338 -> [w358 _]
          tunnel: w346 -> [w357 w371]
          tunnel: [w356 w368] -> w345
          tunnel: w344 -> [w356 _]
          tunnel: [w355 w369] -> w343
          tunnel: w342 -> [w355 _]
          tunnel: [w354 w370] -> w341
          tunnel: w340 -> [w354 w362]
          tunnel: w335 -> [_ w367]
          tunnel: w334 -> [_ w366]
          tunnel: w333 -> [_ w365]
          tunnel: w332 -> [_ w364]
          tunnel: w331 -> [_ w363]
          tunnel: w330 -> [_ w361]
          frame False {
            n114 = call "History_Array_ph.vi"("Current Value"=w357, "Desired Length"=w358, "History In"=w359) -> ("History Out"=w360:dbl[])
          }
          frame True {
            n115 = for {
              tunnel: [w383] -> w370 mode=indexing
              tunnel: [w384] -> w369 mode=indexing
              tunnel: [w385] -> w368 mode=indexing
              tunnel: w367 -> [w376]
              tunnel: w366 -> [w375]
              tunnel: w365 -> [w374] mode=indexing
              tunnel: w364 -> [w386]
              tunnel: w363 -> [w382]
              tunnel: w362 -> [w381]
              tunnel: w361 -> [w373] mode=indexing
              n116 = Search 1D Array(1D array=w382, element=w373) -> (index of element=w380:i32)  [unwired: 1 in]
              n117 = Less Than 0?(x=w380) -> (x < 0?=w378:bool)
              n118 = case shown="True" w378 {
                tunnel: w381 -> [w390 _]
                tunnel: w380 -> [w389 _]
                tunnel: [w388 w391] -> w379
                tunnel: w376 -> [_ w394]
                tunnel: w375 -> [_ w393]
                tunnel: w374 -> [_ w392]
                frame False {
                  n119 = Index Array(array=w390, index=w389) -> (element=w388:dbl)
                }
                frame True {
                  n120 = call "Read_value_of_earlier_Ch.vi"("Desired Ch to Read"=w392, "Ch names"=w393, "Present scan array"=w394) -> ("Value"=w391:dbl)  [unwired: 1 in, 1 out]
                }
              }
              n121 = Not A Number/Path/Refnum?(number/path/refnum=w379) -> (NaN/Path/Refnum?=w377:bool)
              n122 = Select(t=0.0, s=w377, f=w379) -> (s? t:f=w383:dbl)
              n123 = for {
                N: w386 -> [_]
                tunnel: [0.0] -> w385 mode=indexing
                tunnel: [w395] -> w384 mode=indexing
                tunnel: w383 -> [w395]
              }
            }
            n124 = Build Array(w371) -> (w372:dbl[])
          }
        }
        n125 = Array Size(array=w339) -> (size(s)=w336:i32)
        n126 = Equal?(x=w338, y=w336) -> (x = y?=w337:bool)
        n127 = for {
          shift-right: [w352] -> _
          shift-left: 0.0 ("element") -> [w353]
          tunnel: [w352] -> w347 mode=indexing
          tunnel: w339 -> [w351] mode=indexing
          n128 = Add(x=w353, y=w351) -> (x+y=w352:dbl)
        }
      }
      frame #6 {
        # "Temp"
        # "Set"
        n129 = call-poly <vilib>:"Mean.vi"("X"=w401) -> ("mean"=w398:dbl)  [unwired: 1 out]
        n130 = Greater?(x=w418, y=600.0) -> (0:w416:bool)
        n131 = Divide(x="Time (s) before killing heaters when exceeding max power", y=w398) -> (x/y=w397:dbl)
        n132 = To Long Integer(number=w397) -> (32bit integer=w400:i32)
        n133 = for {
          tunnel: w426 -> [w462]
          tunnel: w427 -> [w461]
          tunnel: [w473] -> w434 mode=indexing
          tunnel: w421 -> [w464]
          tunnel: w424 -> [w472]
          tunnel: w433 -> [w466]
          tunnel: [w471] -> w432 mode=indexing
          tunnel: w422 -> [w465]
          tunnel: [w470] -> w431 mode=indexing
          tunnel: w423 -> [w467]
          tunnel: w430 -> [w469] mode=indexing
          tunnel: w429 -> [w460] mode=indexing
          tunnel: w428 -> [w468] mode=indexing
          tunnel: w425 -> [w463]
          tunnel: w420 -> [w456]
          tunnel: w419 -> [w455] mode=indexing
          tunnel: w416 -> [w454]
          tunnel: w415 -> [w453]
          tunnel: w414 -> [w452]
          tunnel: [w451] -> w413 mode=indexing if=w449
          tunnel: [w450] -> w412 mode=indexing if=w449
          tunnel: [w448] -> w411 mode=indexing
          tunnel: [w447] -> w410 mode=indexing
          tunnel: w409 -> [w446]
          tunnel: [w443] -> w408 mode=indexing
          tunnel: [w442] -> w407 mode=indexing
          tunnel: w406 -> [w441]
          tunnel: w405 -> [w440]
          tunnel: [w439] -> w404 mode=indexing
          tunnel: [w438] -> w403 mode=indexing if=w436
          tunnel: w402 -> [w437] mode=indexing
          tunnel: w400 -> [w435]
          i -> [w445]
          # "% Power"
          # "Max Power"
          # "Kd"
          # "Ki"
          # "Kp"
          # "Values Ok"
          # "Integral"
          # "Error"
          # "Error"
          # "Diff"
          n134 = Index Array(array=w446, index=w445) -> (element=w444:i32)
          n135 = Index Array(array=w467, index=w445) -> (element=w459:dbl)
          n136 = Index Array(array=w465, index (row)=w445) -> (element=w457:dbl[])  [unwired: 1 in]
          n137 = Index Array(array=w464, index (row)=w445) -> (element=w458:dbl[])  [unwired: 1 in]
          n138 = stacked-sequence {
            seq-local: [_ _ _ _ _ w621 _ _ _] -> [_ _ _ _ _ _ w652 _ _]
            seq-local: [_ w485 _ _ _ _ _ _ _] -> [_ _ _ _ w600 _ w640 _ _]
            seq-local: [_ w484 _ _ _ _ _ _ _] -> [_ _ _ _ _ w618 _ _ _]
            seq-local: [_ _ _ _ w590 _ _ _ _] -> [_ _ _ _ _ _ w651 _ _]
            seq-local: [_ _ _ _ _ _ w643 _ _] -> [_ _ _ _ _ _ _ w677 w702]
            seq-local: [_ w486 _ _ _ _ _ _ _] -> [_ _ _ _ _ _ w653 _ _]
            seq-local: [_ w478 _ _ _ _ _ _ _] -> [_ _ _ _ _ _ w632 _ _]
            seq-local: [_ w480 _ _ _ _ _ _ _] -> [_ _ w519 w573 _ _ w633 _ _]
            seq-local: [w476 _ _ _ _ _ _ _ _] -> [_ _ _ _ _ _ w644 _ _]
            seq-local: [w475 _ _ _ _ _ _ _ _] -> [_ _ _ _ w593 _ _ _ _]
            seq-local: [w474 _ _ _ _ _ _ _ _] -> [_ _ _ _ _ w616 _ _ _]
            seq-local: [_ _ w516 _ _ _ _ _ _] -> [_ _ _ w582 _ _ w642 _ _]
            seq-local: [_ _ _ _ _ _ "Index To Display" _ _] -> [_ _ _ _ _ _ _ w683 _]
            seq-local: [_ w483 _ _ _ _ _ _ _] -> [_ _ _ _ _ _ _ w681 _]
            seq-local: [_ _ w508 _ _ _ _ _ _] -> [_ _ _ _ _ _ _ _ w704]
            tunnel: w462 -> [_ w498 _ _ _ _ _ w691 _]
            tunnel: w461 -> [_ w497 _ _ _ _ _ w690 _]
            tunnel: [_ w484 _ _ _ _ _ _ _] -> w473
            tunnel: w458 -> [_ w488 _ _ _ _ w654 _ _]
            tunnel: w472 -> [_ _ _ _ w594 _ _ _ _]
            tunnel: w466 -> [_ _ _ _ _ w615 _ _ _]
            tunnel: [_ _ _ _ _ _ w660 _ _] -> w471
            tunnel: w457 -> [_ _ _ w579 _ _ w659 _ _]
            tunnel: [_ _ _ _ w590 _ _ _ _] -> w470
            tunnel: w459 -> [_ _ _ _ w599 _ _ _ _]
            tunnel: w469 -> [_ w489 _ _ _ _ w655 _ _]
            tunnel: w460 -> [_ w490 _ _ _ _ _ _ _]
            tunnel: w468 -> [_ _ w515 w584 _ _ _ w689 _]
            tunnel: w463 -> [_ w487 _ _ _ _ w658 _ _]
            tunnel: w445 -> [_ _ _ _ _ _ w657 _ _]
            tunnel: w456 -> [_ _ _ _ _ _ _ w685 _]
            tunnel: w455 -> [w477 _ _ _ _ _ _ _ _]
            tunnel: w454 -> [_ _ _ w585 _ _ _ _ _]
            tunnel: w453 -> [_ _ w517 _ _ _ _ _ _]
            tunnel: w452 -> [_ _ w518 _ _ _ _ _ _]
            tunnel: [_ _ _ w584 _ _ _ _ _] -> w451
            tunnel: [_ _ _ w583 _ _ _ _ _] -> w449
            tunnel: [_ _ _ w582 _ _ _ _ _] -> w450
            tunnel: [_ _ w513 _ _ _ _ _ _] -> w448
            tunnel: [_ _ _ w575 _ _ _ _ _] -> w447
            tunnel: w444 -> [_ _ _ w576 _ _ _ _ _]
            tunnel: [_ _ _ w573 _ _ _ _ _] -> w443
            tunnel: [_ _ _ _ _ _ _ w678 _] -> w442
            tunnel: w441 -> [_ w482 _ _ _ _ w637 _ _]
            tunnel: w440 -> [_ _ _ _ _ w601 _ _ _]
            tunnel: [_ _ _ _ _ _ _ _ w703] -> w439
            tunnel: [_ _ w505 _ _ _ _ _ _] -> w438
            tunnel: w437 -> [_ _ w505 _ _ _ _ _ _]
            tunnel: [_ _ w504 _ _ _ _ _ _] -> w436
            tunnel: w435 -> [_ _ _ w572 _ _ _ _ _]
            frame #0 {
              n139 = Index Array(array=w477) -> (element #1=w476:dbl, element #2=w475:dbl, element #3=w474:dbl)  [unwired: 3 in]
            }
            frame #1 {
              n140 = call "Read_value_of_earlier_Ch.vi"("Desired Ch to Read"=w489, "Ch names"=w497, "Present scan array"=w498) -> ("Value"=w478:dbl, "Scan comment"=w496:string)  [unwired: 1 in]
              n141 = call "Read_value_of_earlier_Ch.vi"("Desired Ch to Read"=w490, "Ch names"=w497, "Present scan array"=w498) -> ("Value"=w481:dbl, "Scan comment"=w495:string)  [unwired: 1 in]
              n142 = Select(t=w481, s=w482, f=0.0) -> (s? t:f=w480:dbl)
              n143 = Concatenate Strings(w496, w495) -> (w483:string)
              n144 = Not A Number/Path/Refnum?(number/path/refnum=w478) -> (NaN/Path/Refnum?=w493:bool)
              n145 = Not A Number/Path/Refnum?(number/path/refnum=w480) -> (NaN/Path/Refnum?=w492:bool)
              n146 = Subtract(x=w480, y=w478) -> (x-y=w491:dbl)
              n147 = Empty String/Path?(string/path=w483) -> (empty?=w494:bool)
              n148 = Compound Arithmetic op=AND(w494, invert w493, invert w492) -> (w486:bool)
              n149 = case shown="False" w486 {
                tunnel: w488 -> [w499 _]
                tunnel: [w502 w503] -> w485
                tunnel: w491 -> [_ w503]
                frame False {
                  n150 = Array Size(array=w499) -> (size(s)=w500:i32)
                  n151 = Decrement(x=w500) -> (x-1=w501:i32)
                  n152 = Index Array(array=w499, index=w501) -> (element=w502:dbl)
                }
                frame True {
                }
              }
              n153 = call "History_Array_ph.vi"("Current Value"=w485, "Desired Length"=w487, "History In"=w488) -> ("History Out"=w484:dbl[])
            }
            frame #2 {
              n154 = String Length(string="EnFlo_Tunnel:Power:") -> (length=w514:i32)
              n155 = String Subset(string=w515, offset (0)=w514, length (rest)=6 ("length (rest)")) -> (substring=w509:string)
              n156 = Subtract(x=w519, y=w518) -> (x-y=w507:dbl)
              n157 = Multiply(x=w507, y=1.125) -> (x*y=w511:dbl)
              n158 = Increment(x=w511) -> (x+1=w510:dbl)
              n159 = case shown="\"Floor_\"" w509 {
                tunnel: w517 -> [_ w556 w571]
                tunnel: w510 -> [_ w555 w570]
                tunnel: [w529 w544 w561] -> w516
                tunnel: w515 -> [w536 _ _]
                tunnel: w514 -> [w534 _ _]
                tunnel: [w528 FALSE FALSE] -> w513
                tunnel: [w523 w542 2.5 ("kW power capacity")] -> w508
                frame Default {
                  n160 = String Subset(string=w536, offset (0)=w534, length (rest)=10 ("length (rest)")) -> (substring=w526:string)
                  n161 = Equal?(x="Y-ve_Side_", y=w526) -> (x = y?=w524:bool)
                  n162 = Equal?(x="Y+ve_Side_", y=w526) -> (x = y?=w522:bool)
                  n163 = Equal?(x="Source_Hea", y=w526) -> (x = y?=w525:bool)
                  n164 = Compound Arithmetic op=OR(w525, w524, w522) -> (w528:bool)
                  n165 = case shown="False" w524 {
                    tunnel: [w538 3.8 ("kW power capacity")] -> w523
                    tunnel: w522 -> [w540 _]
                    frame False {
                      n166 = Select(t=2.6 ("kW power capacity"), s=w540, f=0.0) -> (s? t:f=w538:dbl)
                    }
                    frame True {
                    }
                  }
                  n167 = Select(t=110.0, s=w528, f=99.0) -> (s? t:f=w529:dbl)
                }
                frame "Inlet_" {
                  w546 = 10.0 ("lower limit")
                  w552 = 100.0  # %
                  w542 = 27.0  # kW power capacity
                  w557 = 1.2  # Density
                  w558 = 0.35  # Area
                  n168 = Compound Arithmetic op=MULTIPLY(w558, w557, w556, w555) -> (w554:dbl)
                  n169 = Divide(x=w554, y=w542) -> (x/y=w553:dbl)
                  n170 = Multiply(x=w553, y=w552) -> (x*y=w545:dbl)
                  n171 = Add(x=w545, y=15.0) -> (x+y=w550:dbl)
                  n172 = In Range and Coerce(upper limit=99.0, x=w550, lower limit=w546) -> (coerced(x)=w547:dbl)  [unwired: 1 out]
                  n173 = Not A Number/Path/Refnum?(number/path/refnum=w547) -> (NaN/Path/Refnum?=w548:bool)
                  n174 = Select(t=w546, s=w548, f=w547) -> (s? t:f=w544:dbl)
                }
                frame "Floor_" {
                  w563 = 10.0 ("lower limit")
                  w569 = 0.75  # Scale
                  n175 = Compound Arithmetic op=MULTIPLY(w569, w571, w570) -> (w562:dbl)
                  n176 = Add(x=w562, y=20.0) -> (x+y=w567:dbl)
                  n177 = In Range and Coerce(upper limit=99.0, x=w567, lower limit=w563) -> (coerced(x)=w564:dbl)  [unwired: 1 out]
                  n178 = Not A Number/Path/Refnum?(number/path/refnum=w564) -> (NaN/Path/Refnum?=w565:bool)
                  n179 = Select(t=w563, s=w565, f=w564) -> (s? t:f=w561:dbl)
                }
              }
              n180 = Greater?(x=w507, y=1.0) -> (0:w504:bool)
            }
            frame #3 {
              n181 = Array Size(array=w579) -> (size(s)=w580:i32)
              n182 = Decrement(x=w580) -> (x-1=w581:i32)
              n183 = Index Array(array=w579, index=w581) -> (element=w578:dbl)
              n184 = Greater?(x=w578, y=w582) -> (0:w577:bool)
              n185 = case shown="True" w577 {
                tunnel: [0 w588] -> w575
                tunnel: w576 -> [_ w587]
                frame False {
                }
                frame True {
                  n186 = Increment(x=w587) -> (x+1=w588:i32)
                }
              }
              n187 = Greater?(x=w575, y=w572) -> (0:w574:bool)
              n188 = Compound Arithmetic op=AND(w574, w577, w585) -> (w583:bool)
            }
            frame #4 {
              w589 = 0.0  # Min
              w598 = 100.0  # Max
              n189 = Multiply(x=w594, y=w600) -> (x*y=w597:dbl)
              n190 = Multiply(x=w597, y=w593) -> (x*y=w596:dbl)
              n191 = Add(x=w596, y=w599) -> (x+y=w595:dbl)
              n192 = In Range and Coerce(upper limit=w598, x=w595, lower limit=w589) -> (coerced(x)=w591:dbl)  [unwired: 1 out]
              n193 = Not A Number/Path/Refnum?(number/path/refnum=w591) -> (NaN/Path/Refnum?=w592:bool)
              n194 = Select(t=w589, s=w592, f=w591) -> (s? t:f=w590:dbl)
            }
            frame #5 {
              n195 = Array Size(array=w615) -> (size(s)=w614:i32)
              n196 = Subtract(x=w614, y=w601) -> (x-y=w617:i32)
              n197 = Array Subset(array=w615, index=w617) -> (w613:dbl[])  [unwired: 1 in]
              n198 = Array Size(array=w613) -> (size(s)=w609:i32)
              n199 = Array Subset(array=w618, index=w617, length=w609) -> (w606:dbl[])
              n200 = Index Array(array=w606, index=0) -> (element=w607:dbl)
              n201 = Array Subset(array=w606, index=1) -> (w604:dbl[])  [unwired: 1 in]
              n202 = for {
                shift-right: [w630] -> _
                shift-left: w607 -> [w631]
                tunnel: w604 -> [w630] mode=indexing
                tunnel: [w626] -> w603
                stop <- w626 stop-if-true
                n203 = Subtract(x=w631, y=w630) -> (x-y=w629:dbl)
                n204 = Absolute Value(x=w629) -> (abs(x)=w628:dbl)
                n205 = Greater?(x=w628, y=3.0) -> (0:w626:bool)
              }
              n206 = call <vilib>:"Linear Fit Coefficients.vi"("Y"=w606, "X"=w613) -> ("slope"=w625:dbl)  [unwired: 3 in, 10 out]
              n207 = Less?(x=w609, y=4) -> (x < y?=w611:bool)
              n208 = Not A Number/Path/Refnum?(number/path/refnum=w625) -> (NaN/Path/Refnum?=w612:bool)
              n209 = Compound Arithmetic op=OR(w611, w612, w603) -> (w610:bool)
              n210 = Select(t=0.0 ("f"), s=w610, f=w625) -> (s? t:f=w623:dbl)
              n211 = Multiply(x=w623, y=w616) -> (x*y=w620:dbl)
              n212 = Not A Number/Path/Refnum?(number/path/refnum=w620) -> (NaN/Path/Refnum?=w622:bool)
              n213 = Select(t=0.0, s=w622, f=w620) -> (s? t:f=w621:dbl)
            }
            frame #6 {
              w634 = 0.0  # Min
              w662 = 100.0  # Max
              n214 = Absolute Value(x=w640) -> (abs(x)=w649:dbl)
              n215 = Greater?(x=w649, y="Proportional Error Deadband") -> (0:w648:bool)
              n216 = Select(t=w640, s=w648, f=0.0) -> (s? t:f=w647:dbl)
              n217 = Multiply(x=w644, y=w647) -> (x*y=w650:dbl)
              n218 = Compound Arithmetic op=ADD(w650, w651, w652) -> (w661:dbl)
              n219 = In Range and Coerce(upper limit=w662, x=w661, lower limit=w634) -> (coerced(x)=w639:dbl)  [unwired: 1 out]
              n220 = Greater Than 0?(x=w632) -> (x > 0?=w636:bool)
              n221 = Not A Number/Path/Refnum?(number/path/refnum=w639) -> (NaN/Path/Refnum?=w638:bool)
              n222 = Compound Arithmetic op=AND(invert w638, w637, w636) -> (w635:bool)
              n223 = Select(t=w639, s=w635, f=w634) -> (s? t:f=w643:dbl)
              n224 = Equal?(x="Index To Display", y=w657) -> (x = y?=w656:bool)
              n225 = case shown="True" w656 {
                tunnel: w650 -> [_ w666]
                tunnel: w643 -> [_ w673]
                tunnel: w652 -> [_ w664]
                tunnel: w651 -> [_ w665]
                tunnel: w655 -> [_ w672]
                tunnel: w633 -> [_ w671]
                tunnel: w632 -> [_ w670]
                tunnel: w654 -> [_ w669]
                tunnel: w653 -> [_ w668]
                tunnel: w642 -> [_ w667]
                tunnel: w640 -> [_ w663]
                frame False {
                }
                frame True {
                  "Control Sum" <- w673
                  "Feedback Temperature" <- w672
                  "Setpoint" <- w671
                  "Current Temp" <- w670
                  "History Out" <- w669
                  "Read Values OK" <- w668
                  "Upper limit on Power" <- w667
                  "Proportional" <- w666
                  "Integral" <- w665
                  "Derivative" <- w664
                  "Error" <- w663
                }
              }
              n226 = call "History_Array_ph.vi"("Current Value"=w643, "Desired Length"=w658, "History In"=w659) -> ("History Out"=w660:dbl[])
            }
            frame #7 {
              n227 = call "Read_value_of_earlier_Ch.vi"("Desired Ch to Read"=w689, "Ch names"=w690, "Present scan array"=w691) -> ("Value"=w688:dbl, "Scan comment"=w679:string)  [unwired: 1 in]
              n228 = Subtract(x=w677, y=w688) -> (x-y=w687:dbl)
              n229 = Absolute Value(x=w687) -> (abs(x)=w686:dbl)
              n230 = Greater?(x=w686, y=w685) -> (0:w675:bool)
              n231 = Equal To 0?(x=w677) -> (x = 0?=w676:bool)
              n232 = Or(x=w676, y=w675) -> (x .or. y?=w674:bool)
              n233 = case shown="True" w674 {
                tunnel: w677 -> [_ w696]
                tunnel: w689 -> [_ w695]
                tunnel: [string[] [] ("Scan Comments") w694] -> w680
                frame False {
                }
                frame True {
                  n234 = Build Array(w695) -> (w697:string[])
                  n235 = Build Array(w696) -> (w698:dbl[])
                  n236 = call "ASYNC_Adam_server.vi"("Values"=w698, "Channel Names"=w697) -> ("Scan Comments"=w694:string[])  [unwired: 1 in, 2 out]
                }
              }
              n237 = feedback-in #3(w683) -> ()
              n238 = feedback #3() -> (w684:i32)  [unwired: 1 in]
              n239 = Not Equal?(x=w683, y=w684) -> (x != y?=w682:bool)
              n240 = case shown="True" w682 {
                frame False {
                }
                frame True {
                  w692 = dbl[] [] ("History Data")
                  n241 = property on="Proportional" class="WFChart (strict)"("History Data"=w692) -> ()  [unwired: 2 in, 2 out]
                  n242 = property on="Integral" class="WFChart (strict)"("History Data"=w692) -> ()  [unwired: 2 in, 2 out]
                  n243 = property on="Derivative" class="WFChart (strict)"("History Data"=w692) -> ()  [unwired: 2 in, 2 out]
                  n244 = property on="Error" class="WFChart (strict)"("History Data"=w692) -> ()  [unwired: 2 in, 2 out]
                }
              }
              n245 = Concatenate Strings(w681, w680, w679) -> (w678:string)
            }
            frame #8 {
              n246 = Subtract(x=w702, y=2.5) -> (x-y=w700:dbl)
              n247 = Less Than 0?(x=w700) -> (x < 0?=w699:bool)
              n248 = case shown="False" w699 {
                tunnel: w704 -> [w709 _]
                tunnel: [w706 0.0] -> w703
                tunnel: w700 -> [w705 _]
                frame False {
                  n249 = Divide(x=w705, y=100.0) -> (x/y=w708:dbl)
                  n250 = Multiply(x=w709, y=w708) -> (x*y=w706:dbl)
                }
                frame True {
                }
              }
            }
          }
        }
      }
      frame #7 {
        # "Check in all the inlet heater Status Channels are correct."
        n251 = while {
          tunnel: w718 -> [w732]
          tunnel: w717 -> [w731]
          tunnel: [w740] -> w716
          tunnel: w715 -> [w739]
          tunnel: w714 -> [w735]
          shift-right: [w736] -> _
          shift-left: _ -> [w737]
          shift-right: [w727] -> _
          shift-left: _ -> [w734]
          shift-right: [w730] -> _
          shift-left: _ -> [w733]
          tunnel: [w726] -> w713
          shift-right: [w725] -> _
          shift-left: _ -> [w724]
          shift-left: _ -> [w723]
          shift-left: _ -> [w722]
          tunnel: w712 -> [w720]
          tunnel: w711 -> [w719]
          stop <- TRUE stop-if-true
          n252 = Unbundle By Name(w739) -> ("Connected Items"=w738:string[])
          n253 = for {
            tunnel: w738 -> [w750] mode=indexing
            tunnel: w735 -> [w767]
            tunnel: [w770] -> w736 mode=indexing
            tunnel: w737 -> [w769]
            tunnel: w734 -> [w765]
            tunnel: w733 -> [w764]
            tunnel: w732 -> [w762]
            tunnel: w731 -> [w761]
            tunnel: [w757] -> w730 mode=indexing
            tunnel: [w758] -> w729 mode=indexing
            tunnel: [w752] -> w728 mode=indexing if=w759
            tunnel: [w743] -> w727 mode=indexing
            tunnel: [w750] -> w726 mode=indexing if=w748
            tunnel: w720 -> [w751]
            tunnel: w719 -> [w742]
            i -> [w766]
            n254 = Search 1D Array(1D array=w767, element=w750) -> (index of element=w760:i32)  [unwired: 1 in]
            n255 = Index Array(array=w769, index=w766) -> (element=w768:i32)
            n256 = Index Array(array=w764, index=w766) -> (element=w756:bool)
            n257 = Index Array(array=w765, index=w766) -> (element=w754:dbl)
            n258 = case shown="Default" w760 {
              tunnel: [w792 0] -> w770
              tunnel: w768 -> [w794 _]
              tunnel: [w791 FALSE] -> w763
              frame Default {
                w795 = 10 ("y")
                n259 = Increment(x=w794) -> (x+1=w793:i32)
                n260 = Greater Or Equal?(x=w794, y=w795) -> (x >= y?=w791:bool)
                n261 = Select(t=w795, s=w791, f=w793) -> (s? t:f=w792:i32)
              }
              frame -1 {
              }
            }
            n262 = Greater Or Equal To 0?(x=w760) -> (x >= 0?=w757:bool)
            n263 = case shown="True" w763 {
              tunnel: w762 -> [_ w786]
              tunnel: w761 -> [_ w785]
              tunnel: w750 -> [w780 w784]
              tunnel: [TRUE w783] -> w758
              tunnel: [w780 w782] -> w752
              frame False {
              }
              frame True {
                n264 = call "Fast_string_Replace.vi"("Replace match with:"="State", "Input String"=w784, "regular expression"="Enable") -> ("Output String"=w782:string)  [unwired: 1 in, 1 out]
                n265 = call "Read_value_of_earlier_Ch.vi"("Desired Ch to Read"=w782, "Ch names"=w785, "Present scan array"=w786) -> ("Value"=w790:dbl)  [unwired: 1 in, 1 out]
                n266 = Greater?(x=w790, y=0.5) -> (0:w783:bool)
              }
            }
            n267 = Equal?(x=w756, y=w757) -> (x = y?=w755:bool)
            n268 = case shown="True" w755 {
              tunnel: w754 -> [w772 w774]
              tunnel: [w771 w773] -> w745
              frame False {
                n269 = Increment(x=w772) -> (x+1=w771:dbl)
              }
              frame True {
                n270 = Greater Than 0?(x=w774) -> (x > 0?=w775:bool)
                n271 = case shown="True" w775 {
                  tunnel: w774 -> [w776 w778]
                  tunnel: [w776 w777] -> w773
                  frame False {
                  }
                  frame True {
                    n272 = Subtract(x=w778, y=0.003) -> (x-y=w777:dbl)
                  }
                }
              }
            }
            n273 = Search 1D Array(1D array=w751, element=w750) -> (index of element=w747:i32)  [unwired: 1 in]
            n274 = Greater Or Equal To 0?(x=w747) -> (x >= 0?=w746:bool)
            n275 = Greater?(x=w745, y=4.2) -> (0:w749:bool)
            n276 = Not(x=w758) -> (.not. x?=w759:bool)
            n277 = And(x=w749, y=w746) -> (x .and. y?=w748:bool)
            n278 = Select(t=w745, s=w742, f=0.0) -> (s? t:f=w743:dbl)
          }
          n279 = And Array Elements(Boolean array=w729) -> (logical AND=w725:bool)
          n280 = Compound Arithmetic op=OR(w725, w724, w723, w722) -> (w721:bool)
          "Heater State Happy" <- w721
          n281 = case shown="False" w721 {
            tunnel: w728 -> [w800 _]
            frame False {
              n282 = for {
                shift-right: [w806] -> w798
                shift-left: "" -> [w808]
                tunnel: w800 -> [w807] mode=indexing
                n283 = Concatenate Strings(w808, w807, "\r\n") -> (w806:string)
              }
              n284 = Format Into String(format string="The State of the following channels is wrong.\n%sThis could be caused by the Policeman tripping out.\nThe EnFlo_Tunnel:Heater:Enable has therefore been set to Zero.", w798) -> (resulting string=w801:string)  [unwired: 2 in, 1 out]
              n285 = call "Server_Emails.vi"("Client Name Contains"="EnFlo_Tunnel", "Message"=w801, "Subject"="Inlet Heater State Error" ("t")) -> ()  [unwired: 2 in, 3 out]
            }
            frame True {
            }
          }
          n286 = Not(x=w721) -> (.not. x?=w740:bool)
        }
      }
      frame #8 {
        n287 = Array Size(array=w815) -> (size(s)=w817:i32)
        n288 = Greater Than 0?(x=w817) -> (x > 0?=w811:bool)
        n289 = And(x=w810, y=w811) -> (x .and. y?=w809:bool)
        n290 = case shown="True" w809 {
          tunnel: w816 -> [_ w824]
          tunnel: w815 -> [_ w825]
          tunnel: [FALSE w823] -> w814
          tunnel: w813 -> [_ w820]
          tunnel: w812 -> [_ w819]
          frame False {
          }
          frame True {
            # "Time"
            # "Dem Vel"
            # "Power"
            # "Setpoint"
            n291 = Get Date/Time In Seconds() -> (seconds since 1Jan1904=w822:timestamp)
            n292 = To Double Precision Float(number=w822) -> (double precision float=w821:dbl)
            n293 = stacked-sequence {
              seq-local: [_ w853 _] -> [_ _ w901]
              seq-local: [w836 _ _] -> [_ w858 _]
              seq-local: [w832 _ _] -> [_ w859 _]
              seq-local: [w830 _ _] -> [_ w857 _]
              seq-local: [w827 _ _] -> [_ w856 _]
              tunnel: w825 -> [w838 w854 _]
              tunnel: w824 -> [_ _ _]
              tunnel: [_ _ w902] -> w823
              tunnel: w821 -> [w837 w855 w900]
              tunnel: w820 -> [_ w852 _]
              tunnel: w819 -> [_ _ _]
              frame #0 {
                w835 = 1 ("index")
                w839 = 1200.0  # Seconds
                w845 = FALSE  # All Active Channels
                n294 = for {
                  tunnel: w838 -> [w849] mode=indexing
                  tunnel: [w848] -> w840 mode=indexing
                  n295 = call "Fast_string_Replace.vi"("Replace match with:"=":Setpoint:" ("regular expression"), "Input String"=w849, "regular expression"=":Power:") -> ("Output String"=w848:string)  [unwired: 2 out]
                }
                n296 = Array Size(array=w838) -> (size(s)=w833:i32)
                n297 = Build Array (concatenate)("EnFlo_Tunnel:Speed:Dem Velocity", w840, w838) -> (w842:string[])
                n298 = call "Channel_Names_and_indicies.vi"("All Active Channels"=w845, "Desired Ch Names"=w842) -> ("Indicies"=w844:i32[])  [unwired: 1 out]
                n299 = Subtract(x=w837, y=w839) -> (x-y=w843:dbl)
                n300 = call "Specified_Channels_server.vi"("End time"=w837, "Start time"=w843, "Clients time"=w837, "Requested channels"=w844) -> ("Output array"=w829:dbl[][], "Centre Times"=w828:dbl[])  [unwired: 1 in, 3 out]
                n301 = Reverse 1D Array(array=w828) -> (reversed array=w827:dbl[])
                n302 = Add(x=w835, y=w833) -> (x+y=w834:i32)
                n303 = for {
                  tunnel: [w847] -> _ mode=indexing
                  tunnel: w829 -> [w847] mode=indexing
                  tunnel: [w846] -> w826 mode=indexing
                  n304 = Reverse 1D Array(array=w847) -> (reversed array=w846:dbl[])
                }
                n305 = Array Subset(array=w826, index (row)=w835, length (row)=w833) -> (w836:dbl[][])  [unwired: 2 in]
                n306 = Array Subset(array=w826, index (row)=w834, length (row)=w833) -> (w832:dbl[][])  [unwired: 2 in]
                n307 = Index Array(array=w826, index (row)=0) -> (element=w830:dbl[])  [unwired: 1 in]
              }
              frame #1 {
                n308 = for {
                  tunnel: w859 -> [w891] mode=indexing
                  tunnel: w858 -> [w889] mode=indexing
                  tunnel: w857 -> [w881]
                  tunnel: w856 -> [w871]
                  tunnel: w855 -> [w870]
                  tunnel: w854 -> [w862] mode=indexing
                  tunnel: [w862] -> w853 mode=indexing if=w860
                  tunnel: w852 -> [w861] mode=indexing
                  n309 = for {
                    tunnel: w891 -> [w899] mode=indexing
                    tunnel: [w897] -> w872
                    tunnel: w861 -> [w896]
                    i -> [w897]
                    stop <- w898 continue-if-true
                    n310 = Greater?(x=w899, y=w896) -> (0:w898:bool)
                  }
                  n311 = Index Array(array=w871, index=w872) -> (element=w869:dbl)
                  n312 = Add(x=10, y=w872) -> (x+y=w882:i32)
                  n313 = Subtract(x=w870, y=w869) -> (x-y=w868:dbl)
                  n314 = Array Subset(array=w889, length=w882) -> (w888:dbl[])  [unwired: 1 in]
                  n315 = Array Subset(array=w881, length=w882) -> (w883:dbl[])  [unwired: 1 in]
                  n316 = Array Max & Min(array=w888) -> (max value=w887:dbl, min value=w886:dbl)  [unwired: 2 out]
                  n317 = Array Max & Min(array=w883) -> (max value=w884:dbl, min value=w885:dbl)  [unwired: 2 out]
                  n318 = Match Pattern(string=w862, regular expression="ve_Side_") -> (offset past match=w866:i32)  [unwired: 1 in, 3 out]
                  n319 = Subtract(x=w887, y=w886) -> (x-y=w880:dbl)
                  n320 = Subtract(x=w884, y=w885) -> (x-y=w878:dbl)
                  n321 = Greater Or Equal To 0?(x=w866) -> (x >= 0?=w865:bool)
                  n322 = Multiply(x=w880, y=4.0) -> (x*y=w875:dbl)
                  n323 = Multiply(x=w878, y=100.0) -> (x*y=w876:dbl)
                  n324 = Max & Min(x=w876, y=w875) -> (max(x,y)=w874:dbl)  [unwired: 1 out]
                  n325 = Add(x=100.0, y=w874) -> (x+y=w864:dbl)
                  n326 = case shown="False" w865 {
                    tunnel: w864 -> [w892 w894]
                    tunnel: [w892 w893] -> w863
                    frame False {
                    }
                    frame True {
                      n327 = Multiply(x=w894, y=15.0) -> (x*y=w893:dbl)
                    }
                  }
                  n328 = Greater?(x=w868, y=w863) -> (0:w860:bool)
                }
              }
              frame #2 {
                n329 = Array Size(array=w901) -> (size(s)=w903:i32)
                n330 = Greater Than 0?(x=w903) -> (x > 0?=w902:bool)
                n331 = case shown="True" w902 {
                  tunnel: w901 -> [_ w905]
                  tunnel: w900 -> [_ w904]
                  frame False {
                  }
                  frame True {
                    n332 = stacked-sequence {
                      seq-local: [w907 _] -> [_ w922]
                      tunnel: w905 -> [w912 w924]
                      tunnel: w904 -> [w911 _]
                      frame #0 {
                        w906 = TRUE  # Contact All clients?
                        n333 = Subtract(x=w911, y=3000.0) -> (x-y=w909:dbl)
                        n334 = call "Channel_Names_and_indicies.vi"("All Active Channels"=FALSE, "Desired Ch Names"=w912) -> ("Indicies"=w915:i32[])  [unwired: 1 out]
                        n335 = call "Specified_Channels_server.vi"("Mode"=Search_mode."Between times", "End time"=w911, "Start time"=w909, "Clients time"=w911, "Requested channels"=w915) -> ("Output array"=w908:dbl[][], "Centre Times"=w916:dbl[])  [unwired: 3 out]
                        n336 = for {
                          tunnel: w916 -> [w919]
                          tunnel: w908 -> [w918] mode=indexing
                          tunnel: [w917] -> w907 mode=indexing
                          n337 = Bundle("Centre Times"=w919, "Output array"=w918) -> (w917:T11)  [unwired: 1 out]
                        }
                        n338 = call "Client_email_addresses.vi"("Contact All clients?"=w906) -> ()  [unwired: 2 in]
                      }
                      frame #1 {
                        n339 = for {
                          shift-right: [w929] -> w920
                          shift-left: "" -> [w932]
                          tunnel: w924 -> [w930] mode=indexing
                          n340 = Concatenate Strings(w932, w930, "\r\n") -> (w929:string)
                        }
                        n341 = Format Into String(format string="The following channels:\n%s\nhave exceeded the maximum anticipated heating power for too long\n\"EnFlo_Tunnel:Heater:Enable\" has therefore been set to 0", w920) -> (resulting string=w925:string)  [unwired: 2 in, 1 out]
                        n342 = call "Email_Attachment_Plot.vi"("X axis name"="Time", "Y axis name"="Power (%)", "XY Graph"=w922, "Series Names"=w924, "message"=w925, "subject ([No Subject])"="Heater Shutdown" ("t")) -> ()  [unwired: 1 out]
                      }
                    }
                  }
                }
              }
            }
          }
        }
      }
      frame #9 {
        n343 = Array Size(array=w937) -> (size(s)=w936:i32)
        n344 = Greater Than 0?(x=w936) -> (x > 0?=w935:bool)
        n345 = And(x=w935, y=w934) -> (x .and. y?=w933:bool)
        n346 = case shown="True" w933 {
          tunnel: w937 -> [_ w940]
          frame False {
          }
          frame True {
            n347 = for {
              shift-right: [w946] -> w938
              shift-left: "" -> [w948]
              tunnel: w940 -> [w947] mode=indexing
              n348 = Concatenate Strings(w948, w947, "\r\n") -> (w946:string)
            }
            n349 = Format Into String(format string="The following channels are turning ON and OFF too frequently:\n%s This could be caused by a 5024 ADAM Module fault. \nThe EnFlo_Tunnel:Heater:Enable has therefore been set ot Zero.", w938) -> (resulting string=w941:string)  [unwired: 2 in, 1 out]
            n350 = call "Server_Emails.vi"("Client Name Contains"="EnFlo_Tunnel", "Message"=w941, "Subject"="Inlet Heater ON/OFF Error" ("t")) -> ()  [unwired: 2 in, 3 out]
          }
        }
      }
      frame #10 {
        n351 = case shown="True" w949 {
          tunnel: w955 -> [_ w979]
          tunnel: [FALSE w978] -> w954
          tunnel: w953 -> [_ w975]
          tunnel: w952 -> [_ w974]
          tunnel: w951 -> [_ w970]
          tunnel: w950 -> [_ w966]
          frame False {
          }
          frame True {
            w965 = 60.0 ("lower limit")
            w976 = "EnFlo_Tunnel:Temp:"
            n352 = Array Max & Min(array=w970) -> (max value=w969:dbl)  [unwired: 3 out]
            n353 = Add(x=w969, y=30.0) -> (x+y=w957:dbl)
            n354 = feedback #4() -> (w958:dbl[])  [unwired: 1 in]
            n355 = Build Array (concatenate)(w957, w958) -> (w963:dbl[])
            n356 = Array Subset(array=w963, length=750) -> (w961:dbl[])  [unwired: 1 in]
            n357 = feedback-in #4(w961) -> ()
            n358 = String Length(string=w976) -> (length=w977:i32)
            n359 = Array Max & Min(array=w961) -> (max value=w960:dbl)  [unwired: 3 out]
            n360 = Not A Number/Path/Refnum?(number/path/refnum=w960) -> (NaN/Path/Refnum?=w967:bool)
            n361 = Select(t=w965, s=w967, f=w960) -> (s? t:f=w964:dbl)
            n362 = In Range and Coerce(upper limit=w966, x=w964, lower limit=w965) -> (coerced(x)=w959:dbl)  [unwired: 1 out]
            n363 = for {
              shift-right: [w985] -> w971
              shift-left: "" -> [w986]
              tunnel: w975 -> [w989] mode=indexing
              tunnel: w977 -> [w990]
              tunnel: w976 -> [w987]
              tunnel: w974 -> [w984] mode=indexing
              tunnel: w959 -> [w983]
              n364 = String Subset(string=w989, length (rest)=w990) -> (substring=w988:string)  [unwired: 1 out]
              n365 = Equal?(x=w988, y=w987) -> (x = y?=w980:bool)
              n366 = Greater?(x=w984, y=w983) -> (0:w981:bool)
              n367 = And(x=w980, y=w981) -> (x .and. y?=w982:bool)
              n368 = case shown="True" w982 {
                tunnel: w989 -> [_ w992]
                tunnel: w986 -> [w991 w994]
                tunnel: [w991 w993] -> w985
                frame False {
                }
                frame True {
                  n369 = Concatenate Strings(w994, w992, "\r\n") -> (w993:string)
                }
              }
            }
            n370 = Empty String/Path?(string/path=w971) -> (empty?=w972:bool)
            n371 = case shown="False" w972 {
              tunnel: w979 -> [_ _]
              tunnel: w959 -> [w997 _]
              tunnel: [TRUE FALSE] -> w978
              tunnel: w971 -> [w996 _]
              frame False {
                n372 = Format Into String(format string="The following channels have reached a temperature of  %.0f deg C\n\n%s\n\n\"EnFlo_Tunnel:Heater:Enable\" has therefore been set to 0", w997, w996) -> (resulting string=w999:string)  [unwired: 2 in, 1 out]
                n373 = call "Server_Emails.vi"("Client Name Contains"="EnFlo_Tunnel", "Message"=w999, "Subject"="Heater Shutdown" ("t")) -> ()  [unwired: 2 in, 3 out]
              }
              frame True {
              }
            }
          }
        }
      }
      frame #11 {
        w1023 = ""
        # "Integer Precision on measure temp\nso that not too many emails are sent"
        n374 = global read "EnFlo_Tunnel_Global.vi" "Minimum Ref Velocity for taking Results"() -> (w1009:dbl)
        n375 = Greater?(x=w1010, y=w1009) -> (0:w1008:bool)
        n376 = Add(x=w1022, y=0.01) -> (x+y=w1020:dbl)
        n377 = Compound Arithmetic op=AND(w1008, w1007, w1004) -> (w1006:bool)
        n378 = for {
          tunnel: w1030 -> [w1074] mode=indexing
          tunnel: w1029 -> [w1043] mode=indexing
          shift-right: [w1075] -> w1024
          shift-left: w1023 -> [w1076]
          tunnel: w1028 -> [w1073] mode=indexing
          tunnel: w1027 -> [w1067] mode=indexing
          tunnel: w1026 -> [w1069]
          tunnel: w1025 -> [w1068]
          shift-right: [w1071] -> w1019
          shift-left: w1023 -> [w1072]
          tunnel: w1020 -> [w1070]
          tunnel: [w1061] -> w1016 mode=indexing
          tunnel: w1015 -> [w1063]
          tunnel: w1014 -> [w1058] mode=indexing
          tunnel: w1013 -> [w1057]
          tunnel: w1012 -> [w1050]
          tunnel: [w1052] -> w1011 mode=indexing
          tunnel: [w1045] -> w1005 mode=indexing
          i -> [w1049]
          n379 = Index Array(array=w1050, index=w1049) -> (element=w1048:i32)
          n380 = Index Array(array=w1063, index=w1049) -> (element=w1060:dbl)
          n381 = call "Mean_fr_NaN_data.vi"("Data"=w1043) -> ("Mean value"=w1044:dbl)  [unwired: 1 out]
          n382 = call "Read_value_of_earlier_Ch.vi"("Desired Ch to Read"=w1067, "Ch names"=w1068, "Present scan array"=w1069) -> ("Value"=w1061:dbl, "Scan comment"=w1046:string)  [unwired: 1 in]
          n383 = Not Equal?(x=w1061, y=w1060) -> (x != y?=w1059:bool)
          n384 = Max & Min(x=w1061, y=w1060) -> (min(x,y)=w1062:dbl)  [unwired: 1 out]
          n385 = Greater?(x=w1044, y=w1070) -> (0:w1065:bool)
          n386 = Increment(x=w1048) -> (x+1=w1055:i32)
          n387 = Less?(x=w1062, y=7.0) -> (x < y?=w1064:bool)
          n388 = Compound Arithmetic op=OR(w1057, w1058, w1065, w1064, w1059) -> (invert w1056:bool)
          n389 = Select(t=w1055, s=w1056, f=0) -> (s? t:f=w1052:i32)
          n390 = Greater?(x=w1052, y=15) -> (0:w1051:bool)
          n391 = case shown="True" w1051 {
            tunnel: w1076 -> [w1079 w1099]
            tunnel: [w1079 w1094] -> w1075
            tunnel: w1074 -> [_ w1098]
            tunnel: w1073 -> [_ w1102]
            tunnel: w1069 -> [_ w1101]
            tunnel: w1068 -> [_ w1100]
            tunnel: w1072 -> [w1078 w1097]
            tunnel: [w1078 w1089] -> w1071
            tunnel: w1061 -> [_ w1081]
            tunnel: ["" w1083] -> w1047
            frame False {
            }
            frame True {
              # "Setpoint"
              # "Current"
              n392 = call "Read_value_of_earlier_Ch.vi"("Desired Ch to Read"=w1102, "Ch names"=w1100, "Present scan array"=w1101) -> ("Value"=w1082:dbl, "Scan comment"=w1083:string)  [unwired: 1 in]
              n393 = Format Into String(format string="%s has a setpoint temp of %.1f and a measured temp of %.1f.\n", initial string=w1099, w1098, w1081, w1082) -> (resulting string=w1095:string)  [unwired: 1 in, 1 out]
              n394 = Subtract(x=w1082, y=w1081) -> (x-y=w1080:dbl)
              n395 = Format Into String(format string="%s has a setpoint temp of %.1f and a measured temp of %.0f.\n", initial string=w1097, w1098, w1081, w1082) -> (resulting string=w1092:string)  [unwired: 1 in, 1 out]
              n396 = Greater?(x=w1081, y=0.02) -> (0:w1085:bool)
              n397 = Greater?(x=w1080, y=0.2) -> (0:w1086:bool)
              n398 = And(x=w1086, y=w1085) -> (x .and. y?=w1084:bool)
              n399 = Select(t=w1095, s=w1084, f="") -> (s? t:f=w1094:string)
              n400 = Select(t=w1092, s=w1084, f="") -> (s? t:f=w1089:string)
            }
          }
          n401 = Concatenate Strings(w1047, w1046) -> (w1045:string)
        }
        n402 = Select(t=w1019, s=w1006, f="") -> (s? t:f=w1017:string)
        n403 = while {
          tunnel: w1024 -> [w1034]
          shift-right: [w1031] -> _
          shift-left: _ -> [w1032]
          tunnel: w1017 -> [w1031]
          stop <- TRUE stop-if-true
          n404 = Not Equal?(x=w1031, y=w1032) -> (x != y?=w1036:bool)
          n405 = Empty String/Path?(string/path=w1031) -> (empty?=w1035:bool)
          n406 = Compound Arithmetic op=AND(w1036, invert w1035) -> (w1033:bool)
          n407 = case shown="True" w1033 {
            tunnel: w1034 -> [_ w1039]
            frame False {
            }
            frame True {
              n408 = Format Into String(format string="The following channels have currently have a zero power demand:\n\n%s\n\n \nPlease check that this is not adversly affecting your experimental conditions.", w1039) -> (resulting string=w1038:string)  [unwired: 2 in, 1 out]
              n409 = call "Server_Emails.vi"("Client Name Contains"="EnFlo_Tunnel", "Message"=w1038, "Subject"="Zero Heater Power Warning" ("t")) -> ()  [unwired: 2 in, 3 out]
            }
          }
        }
      }
      frame #12 {
        n410 = Add Array Elements(numeric array=w1106) -> (sum=w1105:dbl)
        n411 = Build Array("EnFlo_Tunnel:Total Heating:Load (kW)") -> (w1104:string[])
        n412 = Build Array(w1105) -> (w1107:dbl[])
        n413 = call "ASYNC_Adam_server.vi"("Values"=w1107, "Channel Names"=w1104) -> ()  [unwired: 1 in, 3 out]
        n414 = Compound Arithmetic op=OR(w1108, w1112, w1111, w1110) -> (w1109:bool)
        n415 = case shown="True" w1109 {
          tunnel: w1121 -> [_ _]
          tunnel: [string[] [] ("Scan Comments") w1123] -> w1114
          frame False {
          }
          frame True {
            n416 = Build Array("EnFlo_Tunnel:Heater:Enable") -> (w1127:string[])
            n417 = Array Size(array=w1127) -> (size(s)=w1126:i32)
            n418 = Initialize Array(0.0, w1126) -> (w1124:dbl[])
            n419 = call "ASYNC_Adam_server.vi"("Values"=w1124, "Channel Names"=w1127) -> ("Scan Comments"=w1123:string[])  [unwired: 1 in, 2 out]
          }
        }
        n420 = Concatenate Strings(w1120, w1119, w1118, w1117, w1116, w1115, w1114) -> (→"Error String":string)
      }
    }
  }
